vi "BRig_RT__Case_Exp__State_initTrial__LC_Cue__v10.vi"(6 "input_arrTrig":bool[](array[boolean]), 8 "input_dataTrial":u16[][](array[numeric]), 9 "input_dataExp":u16[](array[numeric]), 10 "input_dataLC":u16[](array[numeric]), 11 "input_dataCurrent":u16[](array[numeric])) -> (0 "output_dataTrial":u16[][](array[numeric]), 3 "output_dataCurrent":u16[](array[numeric]), 4 "output_arrTrig":bool[](array[boolean]))   [LabVIEW 2014]
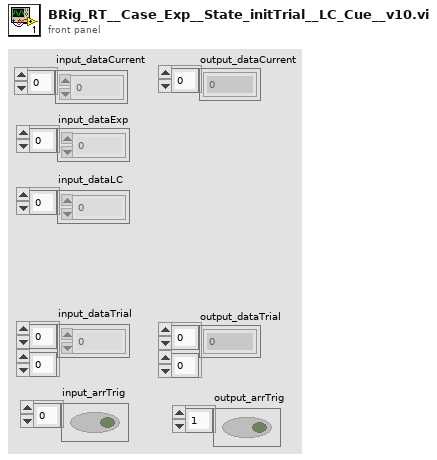
[diagram p1: front panel]
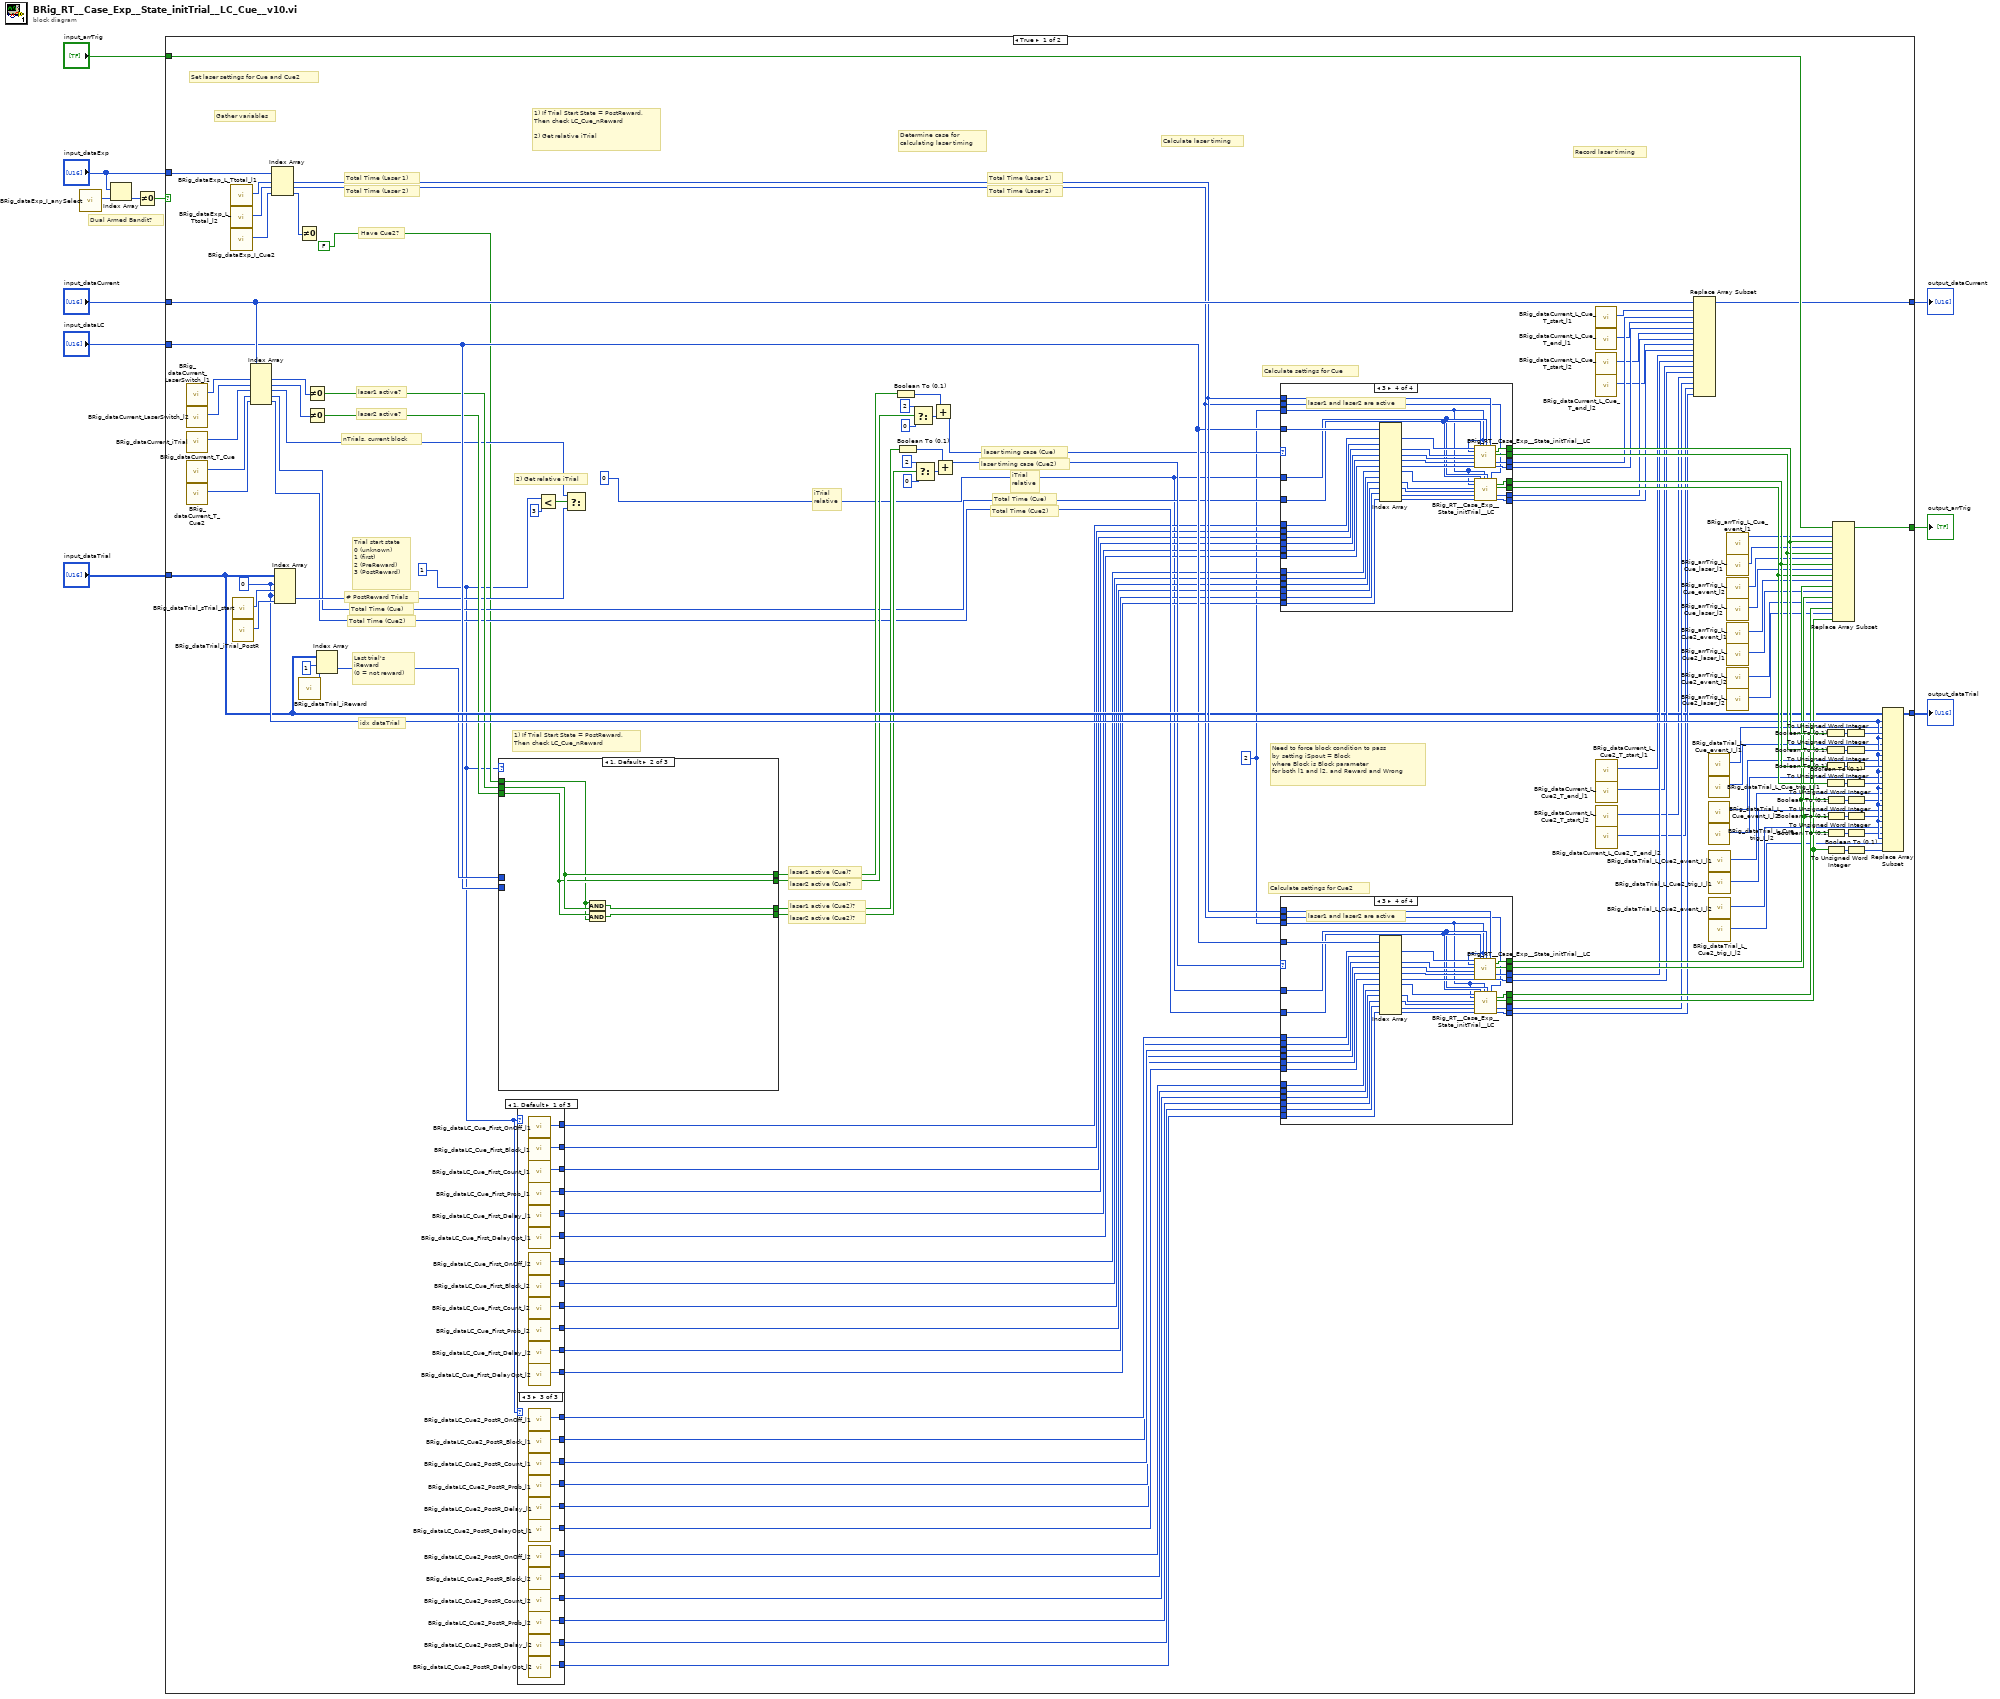
[diagram p0: block diagram]
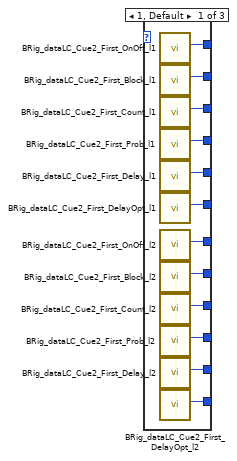
[diagram p2: hidden frame]
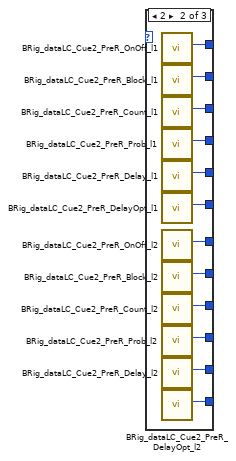
[diagram p3: hidden frame]
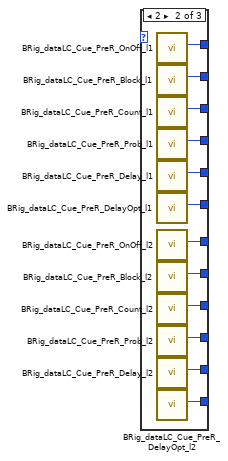
[diagram p4: hidden frame]
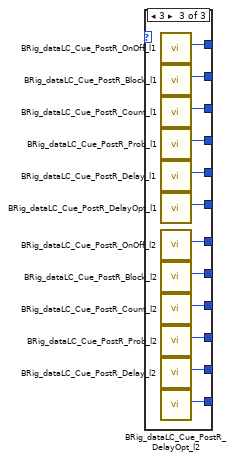
[diagram p5: hidden frame]
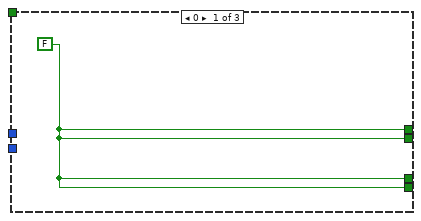
[diagram p6: hidden frame]
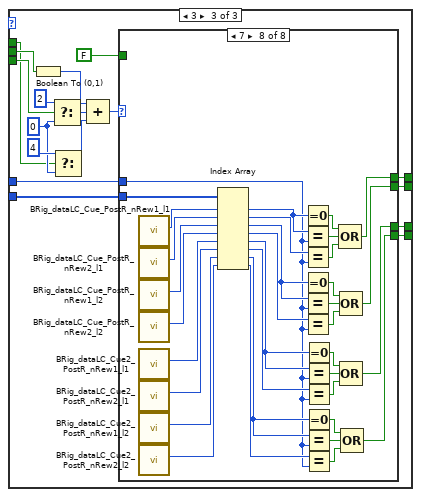
[diagram p7: hidden frame]
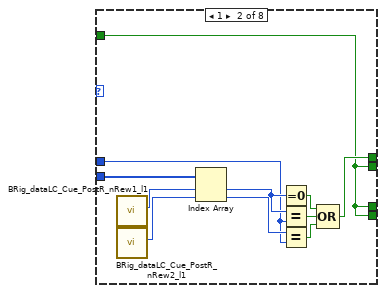
[diagram p9: hidden frame]
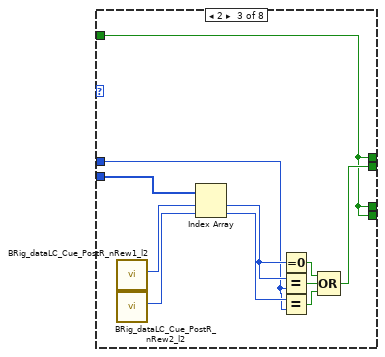
[diagram p10: hidden frame]
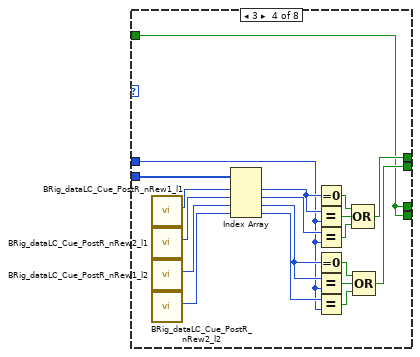
[diagram p11: hidden frame]
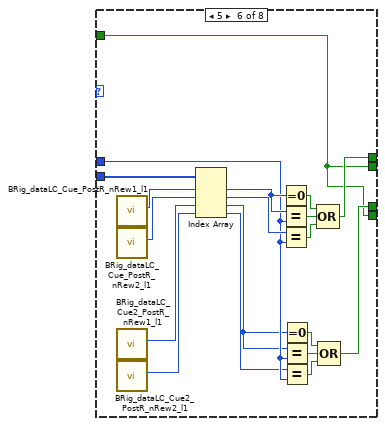
[diagram p13: hidden frame]
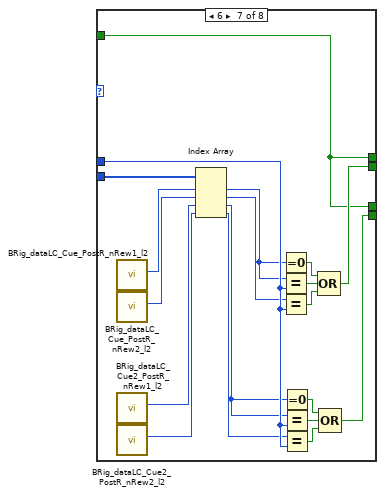
[diagram p14: hidden frame]
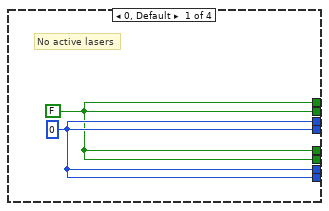
[diagram p15: hidden frame]
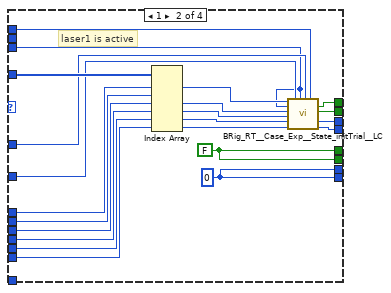
[diagram p16: hidden frame]
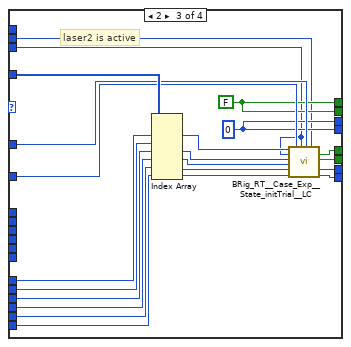
[diagram p17: hidden frame]
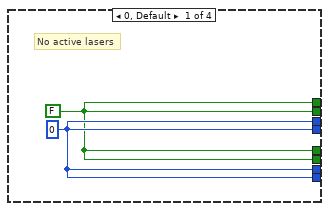
[diagram p18: hidden frame]
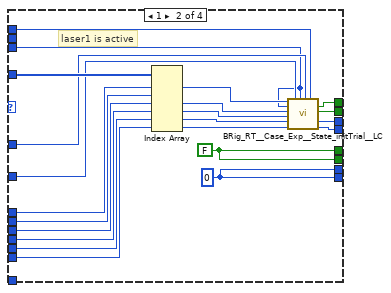
[diagram p19: hidden frame]
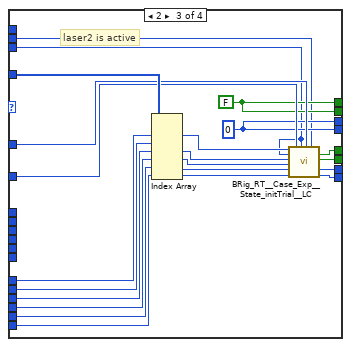
[diagram p20: hidden frame]
diagram:
  # "Dual Armed Bandit?"
  n1 = call "BRig_dataExp_I_anySelect.vi"() -> ("output_I_anySelect"=w4:i32)  [unwired: 11 in]
  n2 = Index Array(array="input_dataExp", index=w4) -> (element=w3:u16)
  n3 = Not Equal To 0?(x=w3) -> (x != 0?=w1:bool)
  n4 = case shown="True" w1 {
    tunnel: "input_arrTrig" -> [w135 w642]
    tunnel: [w134 w641] -> w10
    tunnel: [w121 w628] -> w9
    tunnel: "input_dataCurrent" -> [w120 w627]
    tunnel: [w119 w626] -> w7
    tunnel: "input_dataExp" -> [w112 w619]
    tunnel: "input_dataTrial" -> [w86 w592]
    tunnel: "input_dataLC" -> [w84 w590]
    frame True {
      w12 = u16 2 ("input_sState_start")
      w13 = u16 1
      w14 = u16 0
      w105 = 0
      # "Need to force block condition to pass\nby setting iSpout = Block\nwhere Block is Block parameter\nfor both l1 and l2, and Reward and Wrong"
      # "Record laser timing"
      # "Calculate laser timing"
      # "Total Time (Cue2)"
      # "Total Time (Cue)"
      # "iTrial\nrelative"
      # "Total Time (Laser 2)"
      # "Total Time (Laser 1)"
      # "laser timing case (Cue2)"
      # "Determine case for\ncalculating laser timing"
      # "2) Get relative iTrial"
      # "1) If Trial Start State = PostReward,\nThen check LC_Cue_nReward"
      # "laser2 active (Cue2)?"
      # "laser1 active (Cue2)?"
      # "laser2 active (Cue)?"
      # "laser1 active (Cue)?"
      # "1) If Trial Start State = PostReward,\nThen check LC_Cue_nReward\n\n2) Get relative iTrial"
      # "Gather variables"
      # "Last trial's\niReward\n(0 = not reward)"
      # "nTrials, current block"
      # "idx dataTrial"
      # "Total Time (Cue2)"
      # "Total Time (Cue)"
      # "# PostReward Trials"
      # "Have Cue2?"
      # "Total Time (Laser 2)"
      # "Total Time (Laser 1)"
      # "Calculate settings for Cue2"
      # "Calculate settings for Cue"
      # "Set laser settings for Cue and Cue2"
      # "iTrial\nrelative"
      # "laser timing case (Cue)"
      # "Trial start state\n0 (unknown)\n1 (first)\n2 (PreReward)\n3 (PostReward)"
      # "laser2 active?"
      # "laser1 active?"
      n5 = call "BRig_dataCurrent_LaserSwitch_l1.vi"() -> ("output_LaserSwitch_l1"=w144:i32)  [unwired: 11 in]
      n6 = call "BRig_dataCurrent_LaserSwitch_l2.vi"() -> ("output_LaserSwitch_l2"=w143:i32)  [unwired: 11 in]
      n7 = call "BRig_dataCurrent_iTrial.vi"() -> ("output_iTrial"=w110:i32)  [unwired: 11 in]
      n8 = call "BRig_dataCurrent_T_Cue.vi"() -> ("output_T_Cue"=w67:i32)  [unwired: 11 in]
      n9 = call "BRig_dataCurrent_T_Cue2.vi"() -> ("output_T_Cue2"=w66:i32)  [unwired: 11 in]
      n10 = call "BRig_dataExp_L_Ttotal_l1.vi"() -> ("output_L_Ttotal_l1"=w113:i32)  [unwired: 11 in]
      n11 = call "BRig_dataExp_L_Ttotal_l2.vi"() -> ("output_L_Ttotal_l2"=w114:i32)  [unwired: 11 in]
      n12 = call "BRig_dataExp_I_Cue2.vi"() -> ("output_I_Cue2"=w90:i32)  [unwired: 11 in]
      n13 = call "BRig_dataTrial_sTrial_start.vi"() -> ("output_sTrial_start"=w140:i32)  [unwired: 11 in]
      n14 = call "BRig_dataTrial_iTrial_PostR.vi"() -> ("output_iTrial_PostR"=w111:i32)  [unwired: 11 in]
      n15 = Index Array(array=w120, index #1=w144, index #2=w143, index #3=w110, index #4=w67, index #5=w66) -> (element #1=w142:u16, element #2=w141:u16, element #3=w79:u16, element #4=w65:u16, element #5=w64:u16)
      n16 = Index Array(array=w112, index #1=w113, index #2=w114, index #3=w90) -> (element #1=w100:u16, element #2=w99:u16, element #3=w89:u16)
      n17 = Index Array(array=w86, index (row) #1=w105, index (col) #1=w140, index (row) #2=w105, index (col) #2=w111) -> (element #2=w78:u16)  [unwired: 1 out]
      n18 = Not Equal To 0?(x=w89) -> ()  [unwired: 1 out]
      n19 = call "BRig_dataTrial_iReward.vi"() -> ("output_iReward"=w87:i32)  [unwired: 11 in]
      n20 = Not Equal To 0?(x=w142) -> (x != 0?=w82:bool)
      n21 = Not Equal To 0?(x=w141) -> (x != 0?=w83:bool)
      n22 = Index Array(array=w86, index (row)=1 ("disabled index (row)"), index (col)=w87) -> (element=w85:u16)
      n23 = case shown="1, Default" w13 {
        tunnel: w85 -> [_ _ w231]
        tunnel: w84 -> [_ _ w232]
        tunnel: w83 -> [_ w221 w224]
        tunnel: w82 -> [_ w222 w225]
        tunnel: FALSE -> [_ w220 w223]
        tunnel: [w217 w222 w230] -> w77
        tunnel: [w217 w221 w229] -> w76
        tunnel: [w217 w219 w228] -> w71
        tunnel: [w217 w218 w227] -> w70
        frame 0 {
          w217 = FALSE
        }
        frame 1, Default {
          n24 = And(x=w220, y=w222) -> (x .and. y?=w219:bool)
          n25 = And(x=w221, y=w220) -> (x .and. y?=w218:bool)
        }
        frame 3 {
          w237 = i16 0 ("f")
          n26 = Boolean To (0,1)(Boolean=w225) -> (0, 1=w235:i16)
          n27 = Select(t=i16 2, s=w224, f=w237) -> (s? t:f=w236:i16)
          n28 = Select(t=i16 4, s=w223, f=w237) -> (s? t:f=w234:i16)
          n29 = Compound Arithmetic op=ADD(w235, w236, w234) -> (w233:i16)
          n30 = case shown="7" w233 {
            tunnel: w232 -> [_ w246 w257 w271 _ w296 w317 w344]
            tunnel: w231 -> [_ w245 w256 w270 _ w292 w313 w333]
            tunnel: [w240 w244 w254 w269 w282 w291 w310 w332] -> w230
            tunnel: [w240 w243 w255 w268 w282 w289 w312 w331] -> w229
            tunnel: [w240 w243 w254 w267 w282 w290 w310 w330] -> w228
            tunnel: [w240 w243 w254 w267 w282 w289 w311 w329] -> w227
            tunnel: FALSE -> [w240 w243 w254 w267 w282 w289 w310 _]
            frame 0, Default {
            }
            frame 1 {
              n31 = call "BRig_dataLC_Cue_PostR_nRew1_l1.vi"() -> ("output_Cue_PostR_nRew1_l1"=w241:i32)  [unwired: 11 in]
              n32 = call "BRig_dataLC_Cue_PostR_nRew2_l1.vi"() -> ("output_Cue_PostR_nRew2_l1"=w242:i32)  [unwired: 11 in]
              n33 = Index Array(array=w246, index #1=w241, index #2=w242) -> (element #1=w248:u16, element #2=w247:u16)
              n34 = Equal To 0?(x=w248) -> (x = 0?=w249:bool)
              n35 = Equal?(x=w248, y=w245) -> (x = y?=w250:bool)
              n36 = Equal?(x=w247, y=w245) -> (x = y?=w251:bool)
              n37 = Compound Arithmetic op=OR(w249, w250, w251) -> (w244:bool)
            }
            frame 2 {
              n38 = call "BRig_dataLC_Cue_PostR_nRew1_l2.vi"() -> ("output_Cue_PostR_nRew1_l2"=w252:i32)  [unwired: 11 in]
              n39 = call "BRig_dataLC_Cue_PostR_nRew2_l2.vi"() -> ("output_Cue_PostR_nRew2_l2"=w253:i32)  [unwired: 11 in]
              n40 = Index Array(array=w257, index #1=w252, index #2=w253) -> (element #1=w258:u16, element #2=w259:u16)
              n41 = Equal To 0?(x=w258) -> (x = 0?=w261:bool)
              n42 = Equal?(x=w258, y=w256) -> (x = y?=w260:bool)
              n43 = Equal?(x=w259, y=w256) -> (x = y?=w262:bool)
              n44 = Compound Arithmetic op=OR(w261, w260, w262) -> (w255:bool)
            }
            frame 3 {
              n45 = call "BRig_dataLC_Cue_PostR_nRew1_l1.vi"() -> ("output_Cue_PostR_nRew1_l1"=w263:i32)  [unwired: 11 in]
              n46 = call "BRig_dataLC_Cue_PostR_nRew2_l1.vi"() -> ("output_Cue_PostR_nRew2_l1"=w264:i32)  [unwired: 11 in]
              n47 = call "BRig_dataLC_Cue_PostR_nRew1_l2.vi"() -> ("output_Cue_PostR_nRew1_l2"=w265:i32)  [unwired: 11 in]
              n48 = call "BRig_dataLC_Cue_PostR_nRew2_l2.vi"() -> ("output_Cue_PostR_nRew2_l2"=w266:i32)  [unwired: 11 in]
              n49 = Index Array(array=w271, index #1=w263, index #2=w264, index #3=w265, index #4=w266) -> (element #1=w275:u16, element #2=w274:u16, element #3=w272:u16, element #4=w273:u16)
              n50 = Equal To 0?(x=w275) -> (x = 0?=w276:bool)
              n51 = Equal?(x=w275, y=w270) -> (x = y?=w277:bool)
              n52 = Equal?(x=w274, y=w270) -> (x = y?=w278:bool)
              n53 = Equal To 0?(x=w272) -> (x = 0?=w280:bool)
              n54 = Equal?(x=w272, y=w270) -> (x = y?=w279:bool)
              n55 = Equal?(x=w273, y=w270) -> (x = y?=w281:bool)
              n56 = Compound Arithmetic op=OR(w276, w277, w278) -> (w269:bool)
              n57 = Compound Arithmetic op=OR(w280, w279, w281) -> (w268:bool)
            }
            frame 4 {
            }
            frame 5 {
              n58 = call "BRig_dataLC_Cue_PostR_nRew1_l1.vi"() -> ("output_Cue_PostR_nRew1_l1"=w285:i32)  [unwired: 11 in]
              n59 = call "BRig_dataLC_Cue_PostR_nRew2_l1.vi"() -> ("output_Cue_PostR_nRew2_l1"=w286:i32)  [unwired: 11 in]
              n60 = call "BRig_dataLC_Cue2_PostR_nRew1_l1.vi"() -> ("output_Cue2_PostR_nRew1_l1"=w283:i32)  [unwired: 11 in]
              n61 = call "BRig_dataLC_Cue2_PostR_nRew2_l1.vi"() -> ("output_Cue2_PostR_nRew2_l1"=w284:i32)  [unwired: 11 in]
              n62 = Index Array(array=w296, index #1=w285, index #2=w286, index #3=w283, index #4=w284) -> (element #1=w298:u16, element #2=w297:u16, element #3=w288:u16, element #4=w287:u16)
              n63 = Equal To 0?(x=w298) -> (x = 0?=w299:bool)
              n64 = Equal?(x=w298, y=w292) -> (x = y?=w300:bool)
              n65 = Equal?(x=w297, y=w292) -> (x = y?=w301:bool)
              n66 = Equal To 0?(x=w288) -> (x = 0?=w295:bool)
              n67 = Equal?(x=w288, y=w292) -> (x = y?=w294:bool)
              n68 = Equal?(x=w287, y=w292) -> (x = y?=w293:bool)
              n69 = Compound Arithmetic op=OR(w299, w300, w301) -> (w291:bool)
              n70 = Compound Arithmetic op=OR(w295, w294, w293) -> (w290:bool)
            }
            frame 6 {
              n71 = call "BRig_dataLC_Cue_PostR_nRew1_l2.vi"() -> ("output_Cue_PostR_nRew1_l2"=w305:i32)  [unwired: 11 in]
              n72 = call "BRig_dataLC_Cue_PostR_nRew2_l2.vi"() -> ("output_Cue_PostR_nRew2_l2"=w304:i32)  [unwired: 11 in]
              n73 = call "BRig_dataLC_Cue2_PostR_nRew1_l2.vi"() -> ("output_Cue2_PostR_nRew1_l2"=w303:i32)  [unwired: 11 in]
              n74 = call "BRig_dataLC_Cue2_PostR_nRew2_l2.vi"() -> ("output_Cue2_PostR_nRew2_l2"=w302:i32)  [unwired: 11 in]
              n75 = Index Array(array=w317, index #1=w305, index #2=w304, index #3=w303, index #4=w302) -> (element #1=w309:u16, element #2=w308:u16, element #3=w307:u16, element #4=w306:u16)
              n76 = Equal To 0?(x=w309) -> (x = 0?=w319:bool)
              n77 = Equal?(x=w309, y=w313) -> (x = y?=w318:bool)
              n78 = Equal?(x=w308, y=w313) -> (x = y?=w320:bool)
              n79 = Equal To 0?(x=w307) -> (x = 0?=w315:bool)
              n80 = Equal?(x=w307, y=w313) -> (x = y?=w316:bool)
              n81 = Equal?(x=w306, y=w313) -> (x = y?=w314:bool)
              n82 = Compound Arithmetic op=OR(w319, w318, w320) -> (w312:bool)
              n83 = Compound Arithmetic op=OR(w315, w316, w314) -> (w311:bool)
            }
            frame 7 {
              n84 = call "BRig_dataLC_Cue_PostR_nRew1_l1.vi"() -> ("output_Cue_PostR_nRew1_l1"=w325:i32)  [unwired: 11 in]
              n85 = call "BRig_dataLC_Cue_PostR_nRew2_l1.vi"() -> ("output_Cue_PostR_nRew2_l1"=w326:i32)  [unwired: 11 in]
              n86 = call "BRig_dataLC_Cue_PostR_nRew1_l2.vi"() -> ("output_Cue_PostR_nRew1_l2"=w327:i32)  [unwired: 11 in]
              n87 = call "BRig_dataLC_Cue_PostR_nRew2_l2.vi"() -> ("output_Cue_PostR_nRew2_l2"=w328:i32)  [unwired: 11 in]
              n88 = call "BRig_dataLC_Cue2_PostR_nRew1_l1.vi"() -> ("output_Cue2_PostR_nRew1_l1"=w324:i32)  [unwired: 11 in]
              n89 = call "BRig_dataLC_Cue2_PostR_nRew2_l1.vi"() -> ("output_Cue2_PostR_nRew2_l1"=w323:i32)  [unwired: 11 in]
              n90 = call "BRig_dataLC_Cue2_PostR_nRew1_l2.vi"() -> ("output_Cue2_PostR_nRew1_l2"=w322:i32)  [unwired: 11 in]
              n91 = call "BRig_dataLC_Cue2_PostR_nRew2_l2.vi"() -> ("output_Cue2_PostR_nRew2_l2"=w321:i32)  [unwired: 11 in]
              n92 = Index Array(array=w344, index #1=w325, index #2=w326, index #3=w327, index #4=w328, index #5=w324, index #6=w323, index #7=w322, index #8=w321) -> (element #1=w348:u16, element #2=w347:u16, element #3=w345:u16, element #4=w346:u16, element #5=w337:u16, element #6=w336:u16, element #7=w334:u16, element #8=w335:u16)
              n93 = Equal To 0?(x=w348) -> (x = 0?=w349:bool)
              n94 = Equal?(x=w348, y=w333) -> (x = y?=w350:bool)
              n95 = Equal?(x=w347, y=w333) -> (x = y?=w351:bool)
              n96 = Equal To 0?(x=w345) -> (x = 0?=w353:bool)
              n97 = Equal?(x=w345, y=w333) -> (x = y?=w352:bool)
              n98 = Equal?(x=w346, y=w333) -> (x = y?=w354:bool)
              n99 = Equal To 0?(x=w337) -> (x = 0?=w343:bool)
              n100 = Equal?(x=w337, y=w333) -> (x = y?=w342:bool)
              n101 = Equal?(x=w336, y=w333) -> (x = y?=w341:bool)
              n102 = Equal To 0?(x=w334) -> (x = 0?=w339:bool)
              n103 = Equal?(x=w334, y=w333) -> (x = y?=w340:bool)
              n104 = Equal?(x=w335, y=w333) -> (x = y?=w338:bool)
              n105 = Compound Arithmetic op=OR(w349, w350, w351) -> (w332:bool)
              n106 = Compound Arithmetic op=OR(w353, w352, w354) -> (w331:bool)
              n107 = Compound Arithmetic op=OR(w343, w342, w341) -> (w330:bool)
              n108 = Compound Arithmetic op=OR(w339, w340, w338) -> (w329:bool)
            }
          }
        }
      }
      n109 = case shown="1, Default" w13 {
        tunnel: [w181 w204 w215] -> w52
        tunnel: [w182 w193 w214] -> w53
        tunnel: [w183 w194 w213] -> w54
        tunnel: [w184 w195 w212] -> w55
        tunnel: [w185 w196 w211] -> w56
        tunnel: [w186 w197 w210] -> w57
        tunnel: [w187 w203 w209] -> w58
        tunnel: [w188 w198 w208] -> w59
        tunnel: [w189 w199 w207] -> w60
        tunnel: [w190 w200 w206] -> w61
        tunnel: [w191 w201 w205] -> w62
        tunnel: [w192 w202 w216] -> w63
        frame 1, Default {
          n110 = call "BRig_dataLC_Cue_First_OnOff_l1.vi"() -> ("output_Cue_First_OnOff"=w181:i32)  [unwired: 11 in]
          n111 = call "BRig_dataLC_Cue_First_Block_l1.vi"() -> ("output_Cue_First_Block"=w182:i32)  [unwired: 11 in]
          n112 = call "BRig_dataLC_Cue_First_Count_l1.vi"() -> ("output_Cue_First_Count"=w183:i32)  [unwired: 11 in]
          n113 = call "BRig_dataLC_Cue_First_Prob_l1.vi"() -> ("output_Cue_First_Prob"=w184:i32)  [unwired: 11 in]
          n114 = call "BRig_dataLC_Cue_First_Delay_l1.vi"() -> ("output_Cue_First_Delay"=w185:i32)  [unwired: 11 in]
          n115 = call "BRig_dataLC_Cue_First_DelayOpt_l1.vi"() -> ("output_Cue_First_DelayOpt"=w186:i32)  [unwired: 11 in]
          n116 = call "BRig_dataLC_Cue_First_OnOff_l2.vi"() -> ("output_Cue_First_OnOff_l2"=w187:i32)  [unwired: 11 in]
          n117 = call "BRig_dataLC_Cue_First_Block_l2.vi"() -> ("output_Cue_First_Block_l2"=w188:i32)  [unwired: 11 in]
          n118 = call "BRig_dataLC_Cue_First_Count_l2.vi"() -> ("output_Cue_First_Count_l2"=w189:i32)  [unwired: 11 in]
          n119 = call "BRig_dataLC_Cue_First_Prob_l2.vi"() -> ("output_Cue_First_Prob_l2"=w190:i32)  [unwired: 11 in]
          n120 = call "BRig_dataLC_Cue_First_Delay_l2.vi"() -> ("output_Cue_First_Delay_l2"=w191:i32)  [unwired: 11 in]
          n121 = call "BRig_dataLC_Cue_First_DelayOpt_l2.vi"() -> ("output_Cue_First_DelayOpt_l2"=w192:i32)  [unwired: 11 in]
        }
        frame 2 {
          n122 = call "BRig_dataLC_Cue_PreR_OnOff_l1.vi"() -> ("output_Cue_PreR_OnOff"=w204:i32)  [unwired: 11 in]
          n123 = call "BRig_dataLC_Cue_PreR_Block_l1.vi"() -> ("output_Cue_PreR_Block"=w193:i32)  [unwired: 11 in]
          n124 = call "BRig_dataLC_Cue_PreR_Count_l1.vi"() -> ("output_Cue_PreR_Count"=w194:i32)  [unwired: 11 in]
          n125 = call "BRig_dataLC_Cue_PreR_Prob_l1.vi"() -> ("output_Cue_PreR_Prob"=w195:i32)  [unwired: 11 in]
          n126 = call "BRig_dataLC_Cue_PreR_Delay_l1.vi"() -> ("output_Cue_PreR_Delay"=w196:i32)  [unwired: 11 in]
          n127 = call "BRig_dataLC_Cue_PreR_DelayOpt_l1.vi"() -> ("output_Cue_PreR_DelayOpt"=w197:i32)  [unwired: 11 in]
          n128 = call "BRig_dataLC_Cue_PreR_OnOff_l2.vi"() -> ("output_Cue_PreR_OnOff_l2"=w203:i32)  [unwired: 11 in]
          n129 = call "BRig_dataLC_Cue_PreR_Block_l2.vi"() -> ("output_Cue_PreR_Block_l2"=w198:i32)  [unwired: 11 in]
          n130 = call "BRig_dataLC_Cue_PreR_Count_l2.vi"() -> ("output_Cue_PreR_Count_l2"=w199:i32)  [unwired: 11 in]
          n131 = call "BRig_dataLC_Cue_PreR_Prob_l2.vi"() -> ("output_Cue_PreR_Prob_l2"=w200:i32)  [unwired: 11 in]
          n132 = call "BRig_dataLC_Cue_PreR_Delay_l2.vi"() -> ("output_Cue_PreR_Delay_l2"=w201:i32)  [unwired: 11 in]
          n133 = call "BRig_dataLC_Cue_PreR_DelayOpt_l2.vi"() -> ("output_Cue_PreR_DelayOpt_l2"=w202:i32)  [unwired: 11 in]
        }
        frame 3 {
          n134 = call "BRig_dataLC_Cue_PostR_OnOff_l1.vi"() -> ("output_Cue_PostR_OnOff"=w215:i32)  [unwired: 11 in]
          n135 = call "BRig_dataLC_Cue_PostR_Block_l1.vi"() -> ("output_Cue_PostR_Block"=w214:i32)  [unwired: 11 in]
          n136 = call "BRig_dataLC_Cue_PostR_Count_l1.vi"() -> ("output_Cue_PostR_Count"=w213:i32)  [unwired: 11 in]
          n137 = call "BRig_dataLC_Cue_PostR_Prob_l1.vi"() -> ("output_Cue_PostR_Prob"=w212:i32)  [unwired: 11 in]
          n138 = call "BRig_dataLC_Cue_PostR_Delay_l1.vi"() -> ("output_Cue_PostR_Delay"=w211:i32)  [unwired: 11 in]
          n139 = call "BRig_dataLC_Cue_PostR_DelayOpt_l1.vi"() -> ("output_Cue_PostR_DelayOpt"=w210:i32)  [unwired: 11 in]
          n140 = call "BRig_dataLC_Cue_PostR_OnOff_l2.vi"() -> ("output_Cue_PostR_OnOff_l2"=w209:i32)  [unwired: 11 in]
          n141 = call "BRig_dataLC_Cue_PostR_Block_l2.vi"() -> ("output_Cue_PostR_Block_l2"=w208:i32)  [unwired: 11 in]
          n142 = call "BRig_dataLC_Cue_PostR_Count_l2.vi"() -> ("output_Cue_PostR_Count_l2"=w207:i32)  [unwired: 11 in]
          n143 = call "BRig_dataLC_Cue_PostR_Prob_l2.vi"() -> ("output_Cue_PostR_Prob_l2"=w206:i32)  [unwired: 11 in]
          n144 = call "BRig_dataLC_Cue_PostR_Delay_l2.vi"() -> ("output_Cue_PostR_Delay_l2"=w205:i32)  [unwired: 11 in]
          n145 = call "BRig_dataLC_Cue_PostR_DelayOpt_l2.vi"() -> ("output_Cue_PostR_DelayOpt_l2"=w216:i32)  [unwired: 11 in]
        }
      }
      n146 = case shown="3" w13 {
        tunnel: [w156 w168 w180] -> w51
        tunnel: [w155 w167 w179] -> w50
        tunnel: [w154 w166 w178] -> w49
        tunnel: [w153 w165 w177] -> w48
        tunnel: [w152 w164 w176] -> w47
        tunnel: [w151 w163 w175] -> w46
        tunnel: [w150 w162 w174] -> w45
        tunnel: [w149 w161 w173] -> w44
        tunnel: [w148 w160 w172] -> w43
        tunnel: [w147 w159 w171] -> w42
        tunnel: [w146 w158 w170] -> w41
        tunnel: [w145 w157 w169] -> w40
        frame 1, Default {
          n147 = call "BRig_dataLC_Cue2_First_OnOff_l1.vi"() -> ("output_Cue2_First_OnOff"=w156:i32)  [unwired: 11 in]
          n148 = call "BRig_dataLC_Cue2_First_Block_l1.vi"() -> ("output_Cue2_First_Block"=w155:i32)  [unwired: 11 in]
          n149 = call "BRig_dataLC_Cue2_First_Count_l1.vi"() -> ("output_Cue2_First_Count"=w154:i32)  [unwired: 11 in]
          n150 = call "BRig_dataLC_Cue2_First_Prob_l1.vi"() -> ("output_Cue2_First_Prob"=w153:i32)  [unwired: 11 in]
          n151 = call "BRig_dataLC_Cue2_First_Delay_l1.vi"() -> ("output_Cue2_First_Delay"=w152:i32)  [unwired: 11 in]
          n152 = call "BRig_dataLC_Cue2_First_DelayOpt_l1.vi"() -> ("output_Cue2_First_DelayOpt"=w151:i32)  [unwired: 11 in]
          n153 = call "BRig_dataLC_Cue2_First_OnOff_l2.vi"() -> ("output_Cue2_First_OnOff_l2"=w150:i32)  [unwired: 11 in]
          n154 = call "BRig_dataLC_Cue2_First_Block_l2.vi"() -> ("output_Cue2_First_Block_l2"=w149:i32)  [unwired: 11 in]
          n155 = call "BRig_dataLC_Cue2_First_Count_l2.vi"() -> ("output_Cue2_First_Count_l2"=w148:i32)  [unwired: 11 in]
          n156 = call "BRig_dataLC_Cue2_First_Prob_l2.vi"() -> ("output_Cue2_First_Prob_l2"=w147:i32)  [unwired: 11 in]
          n157 = call "BRig_dataLC_Cue2_First_Delay_l2.vi"() -> ("output_Cue2_First_Delay_l2"=w146:i32)  [unwired: 11 in]
          n158 = call "BRig_dataLC_Cue2_First_DelayOpt_l2.vi"() -> ("output_Cue2_First_DelayOpt_l2"=w145:i32)  [unwired: 11 in]
        }
        frame 2 {
          n159 = call "BRig_dataLC_Cue2_PreR_OnOff_l1.vi"() -> ("output_Cue2_PreR_OnOff"=w168:i32)  [unwired: 11 in]
          n160 = call "BRig_dataLC_Cue2_PreR_Block_l1.vi"() -> ("output_Cue2_PreR_Block"=w167:i32)  [unwired: 11 in]
          n161 = call "BRig_dataLC_Cue2_PreR_Count_l1.vi"() -> ("output_Cue2_PreR_Count"=w166:i32)  [unwired: 11 in]
          n162 = call "BRig_dataLC_Cue2_PreR_Prob_l1.vi"() -> ("output_Cue2_PreR_Prob"=w165:i32)  [unwired: 11 in]
          n163 = call "BRig_dataLC_Cue2_PreR_Delay_l1.vi"() -> ("output_Cue2_PreR_Delay"=w164:i32)  [unwired: 11 in]
          n164 = call "BRig_dataLC_Cue2_PreR_DelayOpt_l1.vi"() -> ("output_Cue2_PreR_DelayOpt"=w163:i32)  [unwired: 11 in]
          n165 = call "BRig_dataLC_Cue2_PreR_OnOff_l2.vi"() -> ("output_Cue2_PreR_OnOff_l2"=w162:i32)  [unwired: 11 in]
          n166 = call "BRig_dataLC_Cue2_PreR_Block_l2.vi"() -> ("output_Cue2_PreR_Block_l2"=w161:i32)  [unwired: 11 in]
          n167 = call "BRig_dataLC_Cue2_PreR_Count_l2.vi"() -> ("output_Cue2_PreR_Count_l2"=w160:i32)  [unwired: 11 in]
          n168 = call "BRig_dataLC_Cue2_PreR_Prob_l2.vi"() -> ("output_Cue2_PreR_Prob_l2"=w159:i32)  [unwired: 11 in]
          n169 = call "BRig_dataLC_Cue2_PreR_Delay_l2.vi"() -> ("output_Cue2_PreR_Delay_l2"=w158:i32)  [unwired: 11 in]
          n170 = call "BRig_dataLC_Cue2_PreR_DelayOpt_l2.vi"() -> ("output_Cue2_PreR_DelayOpt_l2"=w157:i32)  [unwired: 11 in]
        }
        frame 3 {
          n171 = call "BRig_dataLC_Cue2_PostR_OnOff_l1.vi"() -> ("output_Cue2_PostR_OnOff"=w180:i32)  [unwired: 11 in]
          n172 = call "BRig_dataLC_Cue2_PostR_Block_l1.vi"() -> ("output_Cue2_PostR_Block"=w179:i32)  [unwired: 11 in]
          n173 = call "BRig_dataLC_Cue2_PostR_Count_l1.vi"() -> ("output_Cue2_PostR_Count"=w178:i32)  [unwired: 11 in]
          n174 = call "BRig_dataLC_Cue2_PostR_Prob_l1.vi"() -> ("output_Cue2_PostR_Prob"=w177:i32)  [unwired: 11 in]
          n175 = call "BRig_dataLC_Cue2_PostR_Delay_l1.vi"() -> ("output_Cue2_PostR_Delay"=w176:i32)  [unwired: 11 in]
          n176 = call "BRig_dataLC_Cue2_PostR_DelayOpt_l1.vi"() -> ("output_Cue2_PostR_DelayOpt"=w175:i32)  [unwired: 11 in]
          n177 = call "BRig_dataLC_Cue2_PostR_OnOff_l2.vi"() -> ("output_Cue2_PostR_OnOff_l2"=w174:i32)  [unwired: 11 in]
          n178 = call "BRig_dataLC_Cue2_PostR_Block_l2.vi"() -> ("output_Cue2_PostR_Block_l2"=w173:i32)  [unwired: 11 in]
          n179 = call "BRig_dataLC_Cue2_PostR_Count_l2.vi"() -> ("output_Cue2_PostR_Count_l2"=w172:i32)  [unwired: 11 in]
          n180 = call "BRig_dataLC_Cue2_PostR_Prob_l2.vi"() -> ("output_Cue2_PostR_Prob_l2"=w171:i32)  [unwired: 11 in]
          n181 = call "BRig_dataLC_Cue2_PostR_Delay_l2.vi"() -> ("output_Cue2_PostR_Delay_l2"=w170:i32)  [unwired: 11 in]
          n182 = call "BRig_dataLC_Cue2_PostR_DelayOpt_l2.vi"() -> ("output_Cue2_PostR_DelayOpt_l2"=w169:i32)  [unwired: 11 in]
        }
      }
      n183 = Less?(x=w13, y=u16 3) -> (x < y?=w80:bool)
      n184 = Select(t=w79, s=w80, f=w78) -> ()  [unwired: 1 out]
      n185 = Boolean To (0,1)(Boolean=w77) -> (0, 1=w137:i16)
      n186 = Boolean To (0,1)(Boolean=w71) -> (0, 1=w74:i16)
      n187 = Select(t=i16 2, s=w76, f=i16 0) -> (s? t:f=w138:i16)
      n188 = Select(t=i16 2, s=w70, f=i16 0) -> (s? t:f=w73:i16)
      n189 = Add(x=w137, y=w138) -> (x+y=w69:i16)
      n190 = Add(x=w74, y=w73) -> (x+y=w68:i16)
      n191 = case shown="3" w69 {
        tunnel: w84 -> [_ w460 w482 w518]
        tunnel: w12 -> [_ w439 w461 w483]
        tunnel: w65 -> [_ w454 w476 w507]
        tunnel: w14 -> [_ w453 w475 w506]
        tunnel: [w437 w452 w464 w505] -> w129
        tunnel: [w437 w451 w464 w504] -> w126
        tunnel: [w438 w450 w463 w503] -> w118
        tunnel: [w438 w449 w463 w502] -> w117
        tunnel: [w437 w442 w474 w501] -> w122
        tunnel: [w438 w441 w473 w500] -> w116
        tunnel: [w437 w442 w472 w499] -> w124
        tunnel: [w438 w441 w471 w498] -> w115
        tunnel: w52 -> [_ w448 _ w497]
        tunnel: w53 -> [_ w447 _ w496]
        tunnel: w54 -> [_ w446 _ w495]
        tunnel: w55 -> [_ w445 _ w494]
        tunnel: w56 -> [_ w444 _ w493]
        tunnel: w57 -> [_ w443 _ w492]
        tunnel: w58 -> [_ _ w470 w491]
        tunnel: w59 -> [_ _ w469 w490]
        tunnel: w60 -> [_ _ w468 w489]
        tunnel: w61 -> [_ _ w467 w488]
        tunnel: w62 -> [_ _ w466 w487]
        tunnel: w63 -> [_ _ w465 w486]
        tunnel: w100 -> [_ w440 _ w485]
        tunnel: w99 -> [_ _ w462 w484]
        frame 0, Default {
          w438 = u16 0
          w437 = FALSE
          # "No active lasers"
        }
        frame 1 {
          w441 = u16 0
          w442 = FALSE
          # "laser1 is active"
          n192 = Index Array(array=w460, index #1=w448, index #2=w447, index #3=w446, index #4=w445, index #5=w444, index #6=w443) -> (element #1=w459:u16, element #3=w458:u16, element #4=w457:u16, element #5=w456:u16, element #6=w455:u16)  [unwired: 1 out]
          n193 = call "BRig_RT__Case_Exp__State_initTrial__LC.vi"("input_L_OnOff"=w459, "input_L_Block"=w439, "input_L_Count"=w458, "input_L_Prob"=w457, "input_L_Tdelay"=w456, "input_L_delayOpt"=w455, "input_T_state"=w454, "input_iSpout"=w439, "input_iTrial_relative"=w453, "input_L_T"=w440) -> ("output_LC_Event"=w452:bool, "output_LC_Laser"=w451:bool, "output_L_Tstart"=w450:u16, "output_L_Tend"=w449:u16)  [unwired: 6 in]
        }
        frame 2 {
          w463 = u16 0
          w464 = FALSE
          # "laser2 is active"
          n194 = Index Array(array=w482, index #1=w470, index #2=w469, index #3=w468, index #4=w467, index #5=w466, index #6=w465) -> (element #1=w477:u16, element #3=w478:u16, element #4=w479:u16, element #5=w480:u16, element #6=w481:u16)  [unwired: 1 out]
          n195 = call "BRig_RT__Case_Exp__State_initTrial__LC.vi"("input_L_OnOff"=w477, "input_L_Block"=w461, "input_L_Count"=w478, "input_L_Prob"=w479, "input_L_Tdelay"=w480, "input_L_delayOpt"=w481, "input_T_state"=w476, "input_iSpout"=w461, "input_iTrial_relative"=w475, "input_L_T"=w462) -> ("output_LC_Event"=w472:bool, "output_LC_Laser"=w474:bool, "output_L_Tstart"=w473:u16, "output_L_Tend"=w471:u16)  [unwired: 6 in]
        }
        frame 3 {
          # "laser1 and laser2 are active"
          n196 = Index Array(array=w518, index #1=w497, index #2=w496, index #3=w495, index #4=w494, index #5=w493, index #6=w492, index #7=w491, index #8=w490, index #9=w489, index #10=w488, index #11=w487, index #12=w486) -> (element #1=w517:u16, element #3=w516:u16, element #4=w515:u16, element #5=w514:u16, element #6=w513:u16, element #7=w508:u16, element #9=w509:u16, element #10=w510:u16, element #11=w511:u16, element #12=w512:u16)  [unwired: 2 out]
          n197 = call "BRig_RT__Case_Exp__State_initTrial__LC.vi"("input_L_OnOff"=w517, "input_L_Block"=w483, "input_L_Count"=w516, "input_L_Prob"=w515, "input_L_Tdelay"=w514, "input_L_delayOpt"=w513, "input_T_state"=w507, "input_iSpout"=w483, "input_iTrial_relative"=w506, "input_L_T"=w485) -> ("output_LC_Event"=w505:bool, "output_LC_Laser"=w504:bool, "output_L_Tstart"=w503:u16, "output_L_Tend"=w502:u16)  [unwired: 6 in]
          n198 = call "BRig_RT__Case_Exp__State_initTrial__LC.vi"("input_L_OnOff"=w508, "input_L_Block"=w483, "input_L_Count"=w509, "input_L_Prob"=w510, "input_L_Tdelay"=w511, "input_L_delayOpt"=w512, "input_T_state"=w507, "input_iSpout"=w483, "input_iTrial_relative"=w506, "input_L_T"=w484) -> ("output_LC_Event"=w499:bool, "output_LC_Laser"=w501:bool, "output_L_Tstart"=w500:u16, "output_L_Tend"=w498:u16)  [unwired: 6 in]
        }
      }
      n199 = case shown="3" w68 {
        tunnel: w84 -> [_ w378 w400 w436]
        tunnel: w12 -> [_ w357 w379 w401]
        tunnel: w64 -> [_ w372 w394 w425]
        tunnel: w14 -> [_ w371 w393 w424]
        tunnel: [w355 w370 w382 w423] -> w98
        tunnel: [w355 w369 w382 w422] -> w97
        tunnel: [w356 w368 w381 w421] -> w94
        tunnel: [w356 w367 w381 w420] -> w93
        tunnel: [w355 w360 w392 w419] -> w95
        tunnel: [w356 w359 w391 w418] -> w92
        tunnel: [w355 w360 w390 w417] -> w96
        tunnel: [w356 w359 w389 w416] -> w91
        tunnel: w51 -> [_ w366 _ w415]
        tunnel: w50 -> [_ w365 _ w414]
        tunnel: w49 -> [_ w364 _ w413]
        tunnel: w48 -> [_ w363 _ w412]
        tunnel: w47 -> [_ w362 _ w411]
        tunnel: w46 -> [_ w361 _ w410]
        tunnel: w45 -> [_ _ w388 w409]
        tunnel: w44 -> [_ _ w387 w408]
        tunnel: w43 -> [_ _ w386 w407]
        tunnel: w42 -> [_ _ w385 w406]
        tunnel: w41 -> [_ _ w384 w405]
        tunnel: w40 -> [_ _ w383 w404]
        tunnel: w100 -> [_ w358 _ w403]
        tunnel: w99 -> [_ _ w380 w402]
        frame 0, Default {
          w356 = u16 0
          w355 = FALSE
          # "No active lasers"
        }
        frame 1 {
          w359 = u16 0
          w360 = FALSE
          # "laser1 is active"
          n200 = Index Array(array=w378, index #1=w366, index #2=w365, index #3=w364, index #4=w363, index #5=w362, index #6=w361) -> (element #1=w377:u16, element #3=w376:u16, element #4=w375:u16, element #5=w374:u16, element #6=w373:u16)  [unwired: 1 out]
          n201 = call "BRig_RT__Case_Exp__State_initTrial__LC.vi"("input_L_OnOff"=w377, "input_L_Block"=w357, "input_L_Count"=w376, "input_L_Prob"=w375, "input_L_Tdelay"=w374, "input_L_delayOpt"=w373, "input_T_state"=w372, "input_iSpout"=w357, "input_iTrial_relative"=w371, "input_L_T"=w358) -> ("output_LC_Event"=w370:bool, "output_LC_Laser"=w369:bool, "output_L_Tstart"=w368:u16, "output_L_Tend"=w367:u16)  [unwired: 6 in]
        }
        frame 2 {
          w381 = u16 0
          w382 = FALSE
          # "laser2 is active"
          n202 = Index Array(array=w400, index #1=w388, index #2=w387, index #3=w386, index #4=w385, index #5=w384, index #6=w383) -> (element #1=w395:u16, element #3=w396:u16, element #4=w397:u16, element #5=w398:u16, element #6=w399:u16)  [unwired: 1 out]
          n203 = call "BRig_RT__Case_Exp__State_initTrial__LC.vi"("input_L_OnOff"=w395, "input_L_Block"=w379, "input_L_Count"=w396, "input_L_Prob"=w397, "input_L_Tdelay"=w398, "input_L_delayOpt"=w399, "input_T_state"=w394, "input_iSpout"=w379, "input_iTrial_relative"=w393, "input_L_T"=w380) -> ("output_LC_Event"=w390:bool, "output_LC_Laser"=w392:bool, "output_L_Tstart"=w391:u16, "output_L_Tend"=w389:u16)  [unwired: 6 in]
        }
        frame 3 {
          # "laser1 and laser2 are active"
          n204 = Index Array(array=w436, index #1=w415, index #2=w414, index #3=w413, index #4=w412, index #5=w411, index #6=w410, index #7=w409, index #8=w408, index #9=w407, index #10=w406, index #11=w405, index #12=w404) -> (element #1=w435:u16, element #3=w434:u16, element #4=w433:u16, element #5=w432:u16, element #6=w431:u16, element #7=w426:u16, element #9=w427:u16, element #10=w428:u16, element #11=w429:u16, element #12=w430:u16)  [unwired: 2 out]
          n205 = call "BRig_RT__Case_Exp__State_initTrial__LC.vi"("input_L_OnOff"=w435, "input_L_Block"=w401, "input_L_Count"=w434, "input_L_Prob"=w433, "input_L_Tdelay"=w432, "input_L_delayOpt"=w431, "input_T_state"=w425, "input_iSpout"=w401, "input_iTrial_relative"=w424, "input_L_T"=w403) -> ("output_LC_Event"=w423:bool, "output_LC_Laser"=w422:bool, "output_L_Tstart"=w421:u16, "output_L_Tend"=w420:u16)  [unwired: 6 in]
          n206 = call "BRig_RT__Case_Exp__State_initTrial__LC.vi"("input_L_OnOff"=w426, "input_L_Block"=w401, "input_L_Count"=w427, "input_L_Prob"=w428, "input_L_Tdelay"=w429, "input_L_delayOpt"=w430, "input_T_state"=w425, "input_iSpout"=w401, "input_iTrial_relative"=w424, "input_L_T"=w402) -> ("output_LC_Event"=w417:bool, "output_LC_Laser"=w419:bool, "output_L_Tstart"=w418:u16, "output_L_Tend"=w416:u16)  [unwired: 6 in]
        }
      }
      n207 = call "BRig_dataCurrent_L_Cue_T_start_l1.vi"() -> ("outputL_Cue_T_start_l1"=w36:i32)  [unwired: 11 in]
      n208 = call "BRig_dataCurrent_L_Cue_T_end_l1.vi"() -> ("output_L_Cue_T_end_l1"=w37:i32)  [unwired: 11 in]
      n209 = call "BRig_dataCurrent_L_Cue_T_start_l2.vi"() -> ("output_L_Cue_T_start_l2"=w38:i32)  [unwired: 11 in]
      n210 = call "BRig_dataCurrent_L_Cue_T_end_l2.vi"() -> ("output_L_Cue_T_end_l2"=w39:i32)  [unwired: 11 in]
      n211 = call "BRig_dataCurrent_L_Cue2_T_start_l1.vi"() -> ("outputL_Cue2_T_start_l1"=w24:i32)  [unwired: 11 in]
      n212 = call "BRig_dataCurrent_L_Cue2_T_end_l1.vi"() -> ("output_L_Cue2_T_end_l1"=w25:i32)  [unwired: 11 in]
      n213 = call "BRig_dataCurrent_L_Cue2_T_start_l2.vi"() -> ("output_L_Cue2_T_start_l2"=w26:i32)  [unwired: 11 in]
      n214 = call "BRig_dataCurrent_L_Cue2_T_end_l2.vi"() -> ("output_L_Cue2_T_end_l2"=w27:i32)  [unwired: 11 in]
      n215 = Replace Array Subset(array=w120, new element #1=w118, index #1=w36, new element #2=w117, index #2=w37, new element #3=w116, index #3=w38, new element #4=w115, index #4=w39, new element #5=w94, index #5=w24, new element #6=w93, index #6=w25, new element #7=w92, index #7=w26, new element #8=w91, index #8=w27) -> (w119:u16[])
      n216 = call "BRig_dataTrial_L_Cue_event_I_l1.vi"() -> ("output_L_Cue_event_I_l1"=w16:i32)  [unwired: 11 in]
      n217 = call "BRig_dataTrial_L_Cue_trig_I_l1.vi"() -> ("output_L_Cue_trig_I_l1"=w17:i32)  [unwired: 11 in]
      n218 = call "BRig_dataTrial_L_Cue_event_I_l2.vi"() -> ("output_L_Cue_event_I_l2"=w18:i32)  [unwired: 11 in]
      n219 = call "BRig_dataTrial_L_Cue_trig_I_l2.vi"() -> ("output_L_Cue_trig_I_l2"=w19:i32)  [unwired: 11 in]
      n220 = call "BRig_dataTrial_L_Cue2_event_I_l1.vi"() -> ("output_L_Cue2_event_I_l1"=w20:i32)  [unwired: 11 in]
      n221 = call "BRig_dataTrial_L_Cue2_trig_I_l1.vi"() -> ("output_L_Cue2_trig_I_l1"=w21:i32)  [unwired: 11 in]
      n222 = call "BRig_dataTrial_L_Cue2_event_I_l2.vi"() -> ("output_L_Cue2_event_I_l2"=w22:i32)  [unwired: 11 in]
      n223 = call "BRig_dataTrial_L_Cue2_trig_I_l2.vi"() -> ("output_L_Cue2_trig_I_l2"=w23:i32)  [unwired: 11 in]
      n224 = call "BRig_arrTrig_L_Cue_event_l1.vi"() -> ("output_L_Cue_event_l1"=w28:i32)  [unwired: 11 in]
      n225 = call "BRig_arrTrig_L_Cue_laser_l1.vi"() -> ("output_L_Cue_laser_l1"=w29:i32)  [unwired: 11 in]
      n226 = call "BRig_arrTrig_L_Cue_event_l2.vi"() -> ("output_L_Cue_event_l2"=w30:i32)  [unwired: 11 in]
      n227 = call "BRig_arrTrig_L_Cue_laser_l2.vi"() -> ("output_L_Cue_laser_l2"=w31:i32)  [unwired: 11 in]
      n228 = call "BRig_arrTrig_L_Cue2_event_l1.vi"() -> ("output_L_Cue2_event_l1"=w32:i32)  [unwired: 11 in]
      n229 = call "BRig_arrTrig_L_Cue2_laser_l1.vi"() -> ("output_L_Cue2_laser_l1"=w33:i32)  [unwired: 11 in]
      n230 = call "BRig_arrTrig_L_Cue2_event_l2.vi"() -> ("output_L_Cue2_event_l2"=w34:i32)  [unwired: 11 in]
      n231 = call "BRig_arrTrig_L_Cue2_laser_l2.vi"() -> ("output_L_Cue2_laser_l2"=w35:i32)  [unwired: 11 in]
      n232 = Boolean To (0,1)(Boolean=w129) -> (0, 1=w133:i16)
      n233 = Boolean To (0,1)(Boolean=w126) -> (0, 1=w132:i16)
      n234 = Boolean To (0,1)(Boolean=w124) -> (0, 1=w130:i16)
      n235 = Boolean To (0,1)(Boolean=w122) -> (0, 1=w131:i16)
      n236 = Boolean To (0,1)(Boolean=w98) -> (0, 1=w109:i16)
      n237 = Boolean To (0,1)(Boolean=w97) -> (0, 1=w108:i16)
      n238 = Boolean To (0,1)(Boolean=w96) -> (0, 1=w106:i16)
      n239 = Boolean To (0,1)(Boolean=w95) -> (0, 1=w107:i16)
      n240 = Replace Array Subset(array=w135, new element #1=w129, index #1=w28, new element #2=w126, index #2=w29, new element #3=w124, index #3=w30, new element #4=w122, index #4=w31, new element #5=w98, index #5=w32, new element #6=w97, index #6=w33, new element #7=w96, index #7=w34, new element #8=w95, index #8=w35) -> (w134:bool[])
      n241 = To Unsigned Word Integer(number=w133) -> (unsigned 16bit integer=w128:u16)
      n242 = To Unsigned Word Integer(number=w132) -> (unsigned 16bit integer=w127:u16)
      n243 = To Unsigned Word Integer(number=w130) -> (unsigned 16bit integer=w125:u16)
      n244 = To Unsigned Word Integer(number=w131) -> (unsigned 16bit integer=w123:u16)
      n245 = To Unsigned Word Integer(number=w109) -> (unsigned 16bit integer=w104:u16)
      n246 = To Unsigned Word Integer(number=w108) -> (unsigned 16bit integer=w103:u16)
      n247 = To Unsigned Word Integer(number=w106) -> (unsigned 16bit integer=w102:u16)
      n248 = To Unsigned Word Integer(number=w107) -> (unsigned 16bit integer=w101:u16)
      n249 = Replace Array Subset(array=w86, new element #1=w128, index (row) #1=w105, index (col) #1=w16, new element #2=w127, index (row) #2=w105, index (col) #2=w17, new element #3=w125, index (row) #3=w105, index (col) #3=w18, new element #4=w123, index (row) #4=w105, index (col) #4=w19, new element #5=w104, index (row) #5=w105, index (col) #5=w20, new element #6=w103, index (row) #6=w105, index (col) #6=w21, new element #7=w102, index (row) #7=w105, index (col) #7=w22, new element #8=w101, index (row) #8=w105, index (col) #8=w23) -> (w121:u16[][])
    }
    frame False {
      w612 = 0
      # "Record laser timing"
      # "Calculate laser timing"
      # "Total Time (Cue2)"
      # "Total Time (Cue)"
      # "iTrial\nrelative"
      # "Total Time (Laser 2)"
      # "Total Time (Laser 1)"
      # "Current directionality, L or R?"
      # "laser timing case (Cue2)"
      # "Determine case for\ncalculating laser timing"
      # "2) Get relative iTrial"
      # "1) If Trial Start State = PostReward,\nThen check LC_Cue_nReward"
      # "laser2 active (Cue2)?"
      # "laser1 active (Cue2)?"
      # "laser2 active (Cue)?"
      # "laser1 active (Cue)?"
      # "1) If Trial Start State = PostReward,\nThen check LC_Cue_nReward\n\n2) Get relative iTrial"
      # "Gather variables"
      # "Last trial's\niReward\n(0 = not reward)"
      # "nTrials, current block"
      # "idx dataTrial"
      # "Total Time (Cue2)"
      # "Total Time (Cue)"
      # "# PostReward Trials"
      # "Current directionality, L or R?"
      # "Have Cue2?"
      # "Total Time (Laser 2)"
      # "Total Time (Laser 1)"
      # "Calculate settings for Cue2"
      # "Calculate settings for Cue"
      # "Set laser settings for Cue and Cue2"
      # "iTrial\nrelative"
      # "laser timing case (Cue)"
      # "Trial start state\n0 (unknown)\n1 (first)\n2 (PreReward)\n3 (PostReward)"
      # "laser2 active?"
      # "laser1 active?"
      n250 = call "BRig_dataCurrent_iSpout.vi"() -> ("output_iSpout"=w643:i32)  [unwired: 11 in]
      n251 = call "BRig_dataCurrent_LaserSwitch_l1.vi"() -> ("output_LaserSwitch_l1"=w652:i32)  [unwired: 11 in]
      n252 = call "BRig_dataCurrent_LaserSwitch_l2.vi"() -> ("output_LaserSwitch_l2"=w651:i32)  [unwired: 11 in]
      n253 = call "BRig_dataCurrent_iTrial.vi"() -> ("output_iTrial"=w617:i32)  [unwired: 11 in]
      n254 = call "BRig_dataCurrent_T_Cue.vi"() -> ("output_T_Cue"=w571:i32)  [unwired: 11 in]
      n255 = call "BRig_dataCurrent_T_Cue2.vi"() -> ("output_T_Cue2"=w570:i32)  [unwired: 11 in]
      n256 = call "BRig_dataExp_L_Ttotal_l1.vi"() -> ("output_L_Ttotal_l1"=w620:i32)  [unwired: 11 in]
      n257 = call "BRig_dataExp_L_Ttotal_l2.vi"() -> ("output_L_Ttotal_l2"=w621:i32)  [unwired: 11 in]
      n258 = call "BRig_dataExp_I_Cue2.vi"() -> ("output_I_Cue2"=w596:i32)  [unwired: 11 in]
      n259 = call "BRig_dataTrial_sTrial_start.vi"() -> ("output_sTrial_start"=w648:i32)  [unwired: 11 in]
      n260 = call "BRig_dataTrial_iTrial_PostR.vi"() -> ("output_iTrial_PostR"=w618:i32)  [unwired: 11 in]
      n261 = Index Array(array=w627, index #1=w643, index #2=w652, index #3=w651, index #4=w617, index #5=w571, index #6=w570) -> (element #1=w605:u16, element #2=w650:u16, element #3=w649:u16, element #4=w584:u16, element #5=w569:u16, element #6=w568:u16)
      n262 = Index Array(array=w619, index #1=w620, index #2=w621, index #3=w596) -> (element #1=w607:u16, element #2=w606:u16, element #3=w595:u16)
      n263 = Index Array(array=w592, index (row) #1=w612, index (col) #1=w648, index (row) #2=w612, index (col) #2=w618) -> (element #1=w543:u16, element #2=w583:u16)
      n264 = Not Equal To 0?(x=w595) -> (x != 0?=w587:bool)
      n265 = call "BRig_dataTrial_iReward.vi"() -> ("output_iReward"=w593:i32)  [unwired: 11 in]
      n266 = Not Equal To 0?(x=w650) -> (x != 0?=w588:bool)
      n267 = Not Equal To 0?(x=w649) -> (x != 0?=w589:bool)
      n268 = Index Array(array=w592, index (row)=1 ("disabled index (row)"), index (col)=w593) -> (element=w591:u16)
      n269 = case shown="3" w543 {
        tunnel: w591 -> [_ _ w739]
        tunnel: w590 -> [_ _ w740]
        tunnel: w589 -> [_ w729 w732]
        tunnel: w588 -> [_ w730 w733]
        tunnel: w587 -> [_ w728 w731]
        tunnel: [w725 w730 w738] -> w581
        tunnel: [w725 w729 w737] -> w580
        tunnel: [w725 w727 w736] -> w575
        tunnel: [w725 w726 w735] -> w574
        frame 0 {
          w725 = FALSE
        }
        frame 1, Default {
          n270 = And(x=w728, y=w730) -> (x .and. y?=w727:bool)
          n271 = And(x=w729, y=w728) -> (x .and. y?=w726:bool)
        }
        frame 3 {
          w745 = i16 0 ("f")
          n272 = Boolean To (0,1)(Boolean=w733) -> (0, 1=w743:i16)
          n273 = Select(t=i16 2, s=w732, f=w745) -> (s? t:f=w744:i16)
          n274 = Select(t=i16 4, s=w731, f=w745) -> (s? t:f=w742:i16)
          n275 = Compound Arithmetic op=ADD(w743, w744, w742) -> (w741:i16)
          n276 = case shown="7" w741 {
            tunnel: w740 -> [_ w754 w765 w779 _ w804 w825 w852]
            tunnel: w739 -> [_ w753 w764 w778 _ w800 w821 w841]
            tunnel: [w748 w752 w762 w777 w790 w799 w818 w840] -> w738
            tunnel: [w748 w751 w763 w776 w790 w797 w820 w839] -> w737
            tunnel: [w748 w751 w762 w775 w790 w798 w818 w838] -> w736
            tunnel: [w748 w751 w762 w775 w790 w797 w819 w837] -> w735
            tunnel: FALSE -> [w748 w751 w762 w775 w790 w797 w818 _]
            frame 0, Default {
            }
            frame 1 {
              n277 = call "BRig_dataLC_Cue_PostR_nRew1_l1.vi"() -> ("output_Cue_PostR_nRew1_l1"=w749:i32)  [unwired: 11 in]
              n278 = call "BRig_dataLC_Cue_PostR_nRew2_l1.vi"() -> ("output_Cue_PostR_nRew2_l1"=w750:i32)  [unwired: 11 in]
              n279 = Index Array(array=w754, index #1=w749, index #2=w750) -> (element #1=w756:u16, element #2=w755:u16)
              n280 = Equal To 0?(x=w756) -> (x = 0?=w757:bool)
              n281 = Equal?(x=w756, y=w753) -> (x = y?=w758:bool)
              n282 = Equal?(x=w755, y=w753) -> (x = y?=w759:bool)
              n283 = Compound Arithmetic op=OR(w757, w758, w759) -> (w752:bool)
            }
            frame 2 {
              n284 = call "BRig_dataLC_Cue_PostR_nRew1_l2.vi"() -> ("output_Cue_PostR_nRew1_l2"=w760:i32)  [unwired: 11 in]
              n285 = call "BRig_dataLC_Cue_PostR_nRew2_l2.vi"() -> ("output_Cue_PostR_nRew2_l2"=w761:i32)  [unwired: 11 in]
              n286 = Index Array(array=w765, index #1=w760, index #2=w761) -> (element #1=w766:u16, element #2=w767:u16)
              n287 = Equal To 0?(x=w766) -> (x = 0?=w769:bool)
              n288 = Equal?(x=w766, y=w764) -> (x = y?=w768:bool)
              n289 = Equal?(x=w767, y=w764) -> (x = y?=w770:bool)
              n290 = Compound Arithmetic op=OR(w769, w768, w770) -> (w763:bool)
            }
            frame 3 {
              n291 = call "BRig_dataLC_Cue_PostR_nRew1_l1.vi"() -> ("output_Cue_PostR_nRew1_l1"=w771:i32)  [unwired: 11 in]
              n292 = call "BRig_dataLC_Cue_PostR_nRew2_l1.vi"() -> ("output_Cue_PostR_nRew2_l1"=w772:i32)  [unwired: 11 in]
              n293 = call "BRig_dataLC_Cue_PostR_nRew1_l2.vi"() -> ("output_Cue_PostR_nRew1_l2"=w773:i32)  [unwired: 11 in]
              n294 = call "BRig_dataLC_Cue_PostR_nRew2_l2.vi"() -> ("output_Cue_PostR_nRew2_l2"=w774:i32)  [unwired: 11 in]
              n295 = Index Array(array=w779, index #1=w771, index #2=w772, index #3=w773, index #4=w774) -> (element #1=w783:u16, element #2=w782:u16, element #3=w780:u16, element #4=w781:u16)
              n296 = Equal To 0?(x=w783) -> (x = 0?=w784:bool)
              n297 = Equal?(x=w783, y=w778) -> (x = y?=w785:bool)
              n298 = Equal?(x=w782, y=w778) -> (x = y?=w786:bool)
              n299 = Equal To 0?(x=w780) -> (x = 0?=w788:bool)
              n300 = Equal?(x=w780, y=w778) -> (x = y?=w787:bool)
              n301 = Equal?(x=w781, y=w778) -> (x = y?=w789:bool)
              n302 = Compound Arithmetic op=OR(w784, w785, w786) -> (w777:bool)
              n303 = Compound Arithmetic op=OR(w788, w787, w789) -> (w776:bool)
            }
            frame 4 {
            }
            frame 5 {
              n304 = call "BRig_dataLC_Cue_PostR_nRew1_l1.vi"() -> ("output_Cue_PostR_nRew1_l1"=w793:i32)  [unwired: 11 in]
              n305 = call "BRig_dataLC_Cue_PostR_nRew2_l1.vi"() -> ("output_Cue_PostR_nRew2_l1"=w794:i32)  [unwired: 11 in]
              n306 = call "BRig_dataLC_Cue2_PostR_nRew1_l1.vi"() -> ("output_Cue2_PostR_nRew1_l1"=w791:i32)  [unwired: 11 in]
              n307 = call "BRig_dataLC_Cue2_PostR_nRew2_l1.vi"() -> ("output_Cue2_PostR_nRew2_l1"=w792:i32)  [unwired: 11 in]
              n308 = Index Array(array=w804, index #1=w793, index #2=w794, index #3=w791, index #4=w792) -> (element #1=w806:u16, element #2=w805:u16, element #3=w796:u16, element #4=w795:u16)
              n309 = Equal To 0?(x=w806) -> (x = 0?=w807:bool)
              n310 = Equal?(x=w806, y=w800) -> (x = y?=w808:bool)
              n311 = Equal?(x=w805, y=w800) -> (x = y?=w809:bool)
              n312 = Equal To 0?(x=w796) -> (x = 0?=w803:bool)
              n313 = Equal?(x=w796, y=w800) -> (x = y?=w802:bool)
              n314 = Equal?(x=w795, y=w800) -> (x = y?=w801:bool)
              n315 = Compound Arithmetic op=OR(w807, w808, w809) -> (w799:bool)
              n316 = Compound Arithmetic op=OR(w803, w802, w801) -> (w798:bool)
            }
            frame 6 {
              n317 = call "BRig_dataLC_Cue_PostR_nRew1_l2.vi"() -> ("output_Cue_PostR_nRew1_l2"=w813:i32)  [unwired: 11 in]
              n318 = call "BRig_dataLC_Cue_PostR_nRew2_l2.vi"() -> ("output_Cue_PostR_nRew2_l2"=w812:i32)  [unwired: 11 in]
              n319 = call "BRig_dataLC_Cue2_PostR_nRew1_l2.vi"() -> ("output_Cue2_PostR_nRew1_l2"=w811:i32)  [unwired: 11 in]
              n320 = call "BRig_dataLC_Cue2_PostR_nRew2_l2.vi"() -> ("output_Cue2_PostR_nRew2_l2"=w810:i32)  [unwired: 11 in]
              n321 = Index Array(array=w825, index #1=w813, index #2=w812, index #3=w811, index #4=w810) -> (element #1=w817:u16, element #2=w816:u16, element #3=w815:u16, element #4=w814:u16)
              n322 = Equal To 0?(x=w817) -> (x = 0?=w827:bool)
              n323 = Equal?(x=w817, y=w821) -> (x = y?=w826:bool)
              n324 = Equal?(x=w816, y=w821) -> (x = y?=w828:bool)
              n325 = Equal To 0?(x=w815) -> (x = 0?=w823:bool)
              n326 = Equal?(x=w815, y=w821) -> (x = y?=w824:bool)
              n327 = Equal?(x=w814, y=w821) -> (x = y?=w822:bool)
              n328 = Compound Arithmetic op=OR(w827, w826, w828) -> (w820:bool)
              n329 = Compound Arithmetic op=OR(w823, w824, w822) -> (w819:bool)
            }
            frame 7 {
              n330 = call "BRig_dataLC_Cue_PostR_nRew1_l1.vi"() -> ("output_Cue_PostR_nRew1_l1"=w833:i32)  [unwired: 11 in]
              n331 = call "BRig_dataLC_Cue_PostR_nRew2_l1.vi"() -> ("output_Cue_PostR_nRew2_l1"=w834:i32)  [unwired: 11 in]
              n332 = call "BRig_dataLC_Cue_PostR_nRew1_l2.vi"() -> ("output_Cue_PostR_nRew1_l2"=w835:i32)  [unwired: 11 in]
              n333 = call "BRig_dataLC_Cue_PostR_nRew2_l2.vi"() -> ("output_Cue_PostR_nRew2_l2"=w836:i32)  [unwired: 11 in]
              n334 = call "BRig_dataLC_Cue2_PostR_nRew1_l1.vi"() -> ("output_Cue2_PostR_nRew1_l1"=w832:i32)  [unwired: 11 in]
              n335 = call "BRig_dataLC_Cue2_PostR_nRew2_l1.vi"() -> ("output_Cue2_PostR_nRew2_l1"=w831:i32)  [unwired: 11 in]
              n336 = call "BRig_dataLC_Cue2_PostR_nRew1_l2.vi"() -> ("output_Cue2_PostR_nRew1_l2"=w830:i32)  [unwired: 11 in]
              n337 = call "BRig_dataLC_Cue2_PostR_nRew2_l2.vi"() -> ("output_Cue2_PostR_nRew2_l2"=w829:i32)  [unwired: 11 in]
              n338 = Index Array(array=w852, index #1=w833, index #2=w834, index #3=w835, index #4=w836, index #5=w832, index #6=w831, index #7=w830, index #8=w829) -> (element #1=w856:u16, element #2=w855:u16, element #3=w853:u16, element #4=w854:u16, element #5=w845:u16, element #6=w844:u16, element #7=w842:u16, element #8=w843:u16)
              n339 = Equal To 0?(x=w856) -> (x = 0?=w857:bool)
              n340 = Equal?(x=w856, y=w841) -> (x = y?=w858:bool)
              n341 = Equal?(x=w855, y=w841) -> (x = y?=w859:bool)
              n342 = Equal To 0?(x=w853) -> (x = 0?=w861:bool)
              n343 = Equal?(x=w853, y=w841) -> (x = y?=w860:bool)
              n344 = Equal?(x=w854, y=w841) -> (x = y?=w862:bool)
              n345 = Equal To 0?(x=w845) -> (x = 0?=w851:bool)
              n346 = Equal?(x=w845, y=w841) -> (x = y?=w850:bool)
              n347 = Equal?(x=w844, y=w841) -> (x = y?=w849:bool)
              n348 = Equal To 0?(x=w842) -> (x = 0?=w847:bool)
              n349 = Equal?(x=w842, y=w841) -> (x = y?=w848:bool)
              n350 = Equal?(x=w843, y=w841) -> (x = y?=w846:bool)
              n351 = Compound Arithmetic op=OR(w857, w858, w859) -> (w840:bool)
              n352 = Compound Arithmetic op=OR(w861, w860, w862) -> (w839:bool)
              n353 = Compound Arithmetic op=OR(w851, w850, w849) -> (w838:bool)
              n354 = Compound Arithmetic op=OR(w847, w848, w846) -> (w837:bool)
            }
          }
        }
      }
      n355 = case shown="1, Default" w543 {
        tunnel: [w689 w712 w723] -> w556
        tunnel: [w690 w701 w722] -> w557
        tunnel: [w691 w702 w721] -> w558
        tunnel: [w692 w703 w720] -> w559
        tunnel: [w693 w704 w719] -> w560
        tunnel: [w694 w705 w718] -> w561
        tunnel: [w695 w711 w717] -> w562
        tunnel: [w696 w706 w716] -> w563
        tunnel: [w697 w707 w715] -> w564
        tunnel: [w698 w708 w714] -> w565
        tunnel: [w699 w709 w713] -> w566
        tunnel: [w700 w710 w724] -> w567
        frame 1, Default {
          n356 = call "BRig_dataLC_Cue_First_OnOff_l1.vi"() -> ("output_Cue_First_OnOff"=w689:i32)  [unwired: 11 in]
          n357 = call "BRig_dataLC_Cue_First_Block_l1.vi"() -> ("output_Cue_First_Block"=w690:i32)  [unwired: 11 in]
          n358 = call "BRig_dataLC_Cue_First_Count_l1.vi"() -> ("output_Cue_First_Count"=w691:i32)  [unwired: 11 in]
          n359 = call "BRig_dataLC_Cue_First_Prob_l1.vi"() -> ("output_Cue_First_Prob"=w692:i32)  [unwired: 11 in]
          n360 = call "BRig_dataLC_Cue_First_Delay_l1.vi"() -> ("output_Cue_First_Delay"=w693:i32)  [unwired: 11 in]
          n361 = call "BRig_dataLC_Cue_First_DelayOpt_l1.vi"() -> ("output_Cue_First_DelayOpt"=w694:i32)  [unwired: 11 in]
          n362 = call "BRig_dataLC_Cue_First_OnOff_l2.vi"() -> ("output_Cue_First_OnOff_l2"=w695:i32)  [unwired: 11 in]
          n363 = call "BRig_dataLC_Cue_First_Block_l2.vi"() -> ("output_Cue_First_Block_l2"=w696:i32)  [unwired: 11 in]
          n364 = call "BRig_dataLC_Cue_First_Count_l2.vi"() -> ("output_Cue_First_Count_l2"=w697:i32)  [unwired: 11 in]
          n365 = call "BRig_dataLC_Cue_First_Prob_l2.vi"() -> ("output_Cue_First_Prob_l2"=w698:i32)  [unwired: 11 in]
          n366 = call "BRig_dataLC_Cue_First_Delay_l2.vi"() -> ("output_Cue_First_Delay_l2"=w699:i32)  [unwired: 11 in]
          n367 = call "BRig_dataLC_Cue_First_DelayOpt_l2.vi"() -> ("output_Cue_First_DelayOpt_l2"=w700:i32)  [unwired: 11 in]
        }
        frame 2 {
          n368 = call "BRig_dataLC_Cue_PreR_OnOff_l1.vi"() -> ("output_Cue_PreR_OnOff"=w712:i32)  [unwired: 11 in]
          n369 = call "BRig_dataLC_Cue_PreR_Block_l1.vi"() -> ("output_Cue_PreR_Block"=w701:i32)  [unwired: 11 in]
          n370 = call "BRig_dataLC_Cue_PreR_Count_l1.vi"() -> ("output_Cue_PreR_Count"=w702:i32)  [unwired: 11 in]
          n371 = call "BRig_dataLC_Cue_PreR_Prob_l1.vi"() -> ("output_Cue_PreR_Prob"=w703:i32)  [unwired: 11 in]
          n372 = call "BRig_dataLC_Cue_PreR_Delay_l1.vi"() -> ("output_Cue_PreR_Delay"=w704:i32)  [unwired: 11 in]
          n373 = call "BRig_dataLC_Cue_PreR_DelayOpt_l1.vi"() -> ("output_Cue_PreR_DelayOpt"=w705:i32)  [unwired: 11 in]
          n374 = call "BRig_dataLC_Cue_PreR_OnOff_l2.vi"() -> ("output_Cue_PreR_OnOff_l2"=w711:i32)  [unwired: 11 in]
          n375 = call "BRig_dataLC_Cue_PreR_Block_l2.vi"() -> ("output_Cue_PreR_Block_l2"=w706:i32)  [unwired: 11 in]
          n376 = call "BRig_dataLC_Cue_PreR_Count_l2.vi"() -> ("output_Cue_PreR_Count_l2"=w707:i32)  [unwired: 11 in]
          n377 = call "BRig_dataLC_Cue_PreR_Prob_l2.vi"() -> ("output_Cue_PreR_Prob_l2"=w708:i32)  [unwired: 11 in]
          n378 = call "BRig_dataLC_Cue_PreR_Delay_l2.vi"() -> ("output_Cue_PreR_Delay_l2"=w709:i32)  [unwired: 11 in]
          n379 = call "BRig_dataLC_Cue_PreR_DelayOpt_l2.vi"() -> ("output_Cue_PreR_DelayOpt_l2"=w710:i32)  [unwired: 11 in]
        }
        frame 3 {
          n380 = call "BRig_dataLC_Cue_PostR_OnOff_l1.vi"() -> ("output_Cue_PostR_OnOff"=w723:i32)  [unwired: 11 in]
          n381 = call "BRig_dataLC_Cue_PostR_Block_l1.vi"() -> ("output_Cue_PostR_Block"=w722:i32)  [unwired: 11 in]
          n382 = call "BRig_dataLC_Cue_PostR_Count_l1.vi"() -> ("output_Cue_PostR_Count"=w721:i32)  [unwired: 11 in]
          n383 = call "BRig_dataLC_Cue_PostR_Prob_l1.vi"() -> ("output_Cue_PostR_Prob"=w720:i32)  [unwired: 11 in]
          n384 = call "BRig_dataLC_Cue_PostR_Delay_l1.vi"() -> ("output_Cue_PostR_Delay"=w719:i32)  [unwired: 11 in]
          n385 = call "BRig_dataLC_Cue_PostR_DelayOpt_l1.vi"() -> ("output_Cue_PostR_DelayOpt"=w718:i32)  [unwired: 11 in]
          n386 = call "BRig_dataLC_Cue_PostR_OnOff_l2.vi"() -> ("output_Cue_PostR_OnOff_l2"=w717:i32)  [unwired: 11 in]
          n387 = call "BRig_dataLC_Cue_PostR_Block_l2.vi"() -> ("output_Cue_PostR_Block_l2"=w716:i32)  [unwired: 11 in]
          n388 = call "BRig_dataLC_Cue_PostR_Count_l2.vi"() -> ("output_Cue_PostR_Count_l2"=w715:i32)  [unwired: 11 in]
          n389 = call "BRig_dataLC_Cue_PostR_Prob_l2.vi"() -> ("output_Cue_PostR_Prob_l2"=w714:i32)  [unwired: 11 in]
          n390 = call "BRig_dataLC_Cue_PostR_Delay_l2.vi"() -> ("output_Cue_PostR_Delay_l2"=w713:i32)  [unwired: 11 in]
          n391 = call "BRig_dataLC_Cue_PostR_DelayOpt_l2.vi"() -> ("output_Cue_PostR_DelayOpt_l2"=w724:i32)  [unwired: 11 in]
        }
      }
      n392 = case shown="3" w543 {
        tunnel: [w664 w676 w688] -> w555
        tunnel: [w663 w675 w687] -> w554
        tunnel: [w662 w674 w686] -> w553
        tunnel: [w661 w673 w685] -> w552
        tunnel: [w660 w672 w684] -> w551
        tunnel: [w659 w671 w683] -> w550
        tunnel: [w658 w670 w682] -> w549
        tunnel: [w657 w669 w681] -> w548
        tunnel: [w656 w668 w680] -> w547
        tunnel: [w655 w667 w679] -> w546
        tunnel: [w654 w666 w678] -> w545
        tunnel: [w653 w665 w677] -> w544
        frame 1, Default {
          n393 = call "BRig_dataLC_Cue2_First_OnOff_l1.vi"() -> ("output_Cue2_First_OnOff"=w664:i32)  [unwired: 11 in]
          n394 = call "BRig_dataLC_Cue2_First_Block_l1.vi"() -> ("output_Cue2_First_Block"=w663:i32)  [unwired: 11 in]
          n395 = call "BRig_dataLC_Cue2_First_Count_l1.vi"() -> ("output_Cue2_First_Count"=w662:i32)  [unwired: 11 in]
          n396 = call "BRig_dataLC_Cue2_First_Prob_l1.vi"() -> ("output_Cue2_First_Prob"=w661:i32)  [unwired: 11 in]
          n397 = call "BRig_dataLC_Cue2_First_Delay_l1.vi"() -> ("output_Cue2_First_Delay"=w660:i32)  [unwired: 11 in]
          n398 = call "BRig_dataLC_Cue2_First_DelayOpt_l1.vi"() -> ("output_Cue2_First_DelayOpt"=w659:i32)  [unwired: 11 in]
          n399 = call "BRig_dataLC_Cue2_First_OnOff_l2.vi"() -> ("output_Cue2_First_OnOff_l2"=w658:i32)  [unwired: 11 in]
          n400 = call "BRig_dataLC_Cue2_First_Block_l2.vi"() -> ("output_Cue2_First_Block_l2"=w657:i32)  [unwired: 11 in]
          n401 = call "BRig_dataLC_Cue2_First_Count_l2.vi"() -> ("output_Cue2_First_Count_l2"=w656:i32)  [unwired: 11 in]
          n402 = call "BRig_dataLC_Cue2_First_Prob_l2.vi"() -> ("output_Cue2_First_Prob_l2"=w655:i32)  [unwired: 11 in]
          n403 = call "BRig_dataLC_Cue2_First_Delay_l2.vi"() -> ("output_Cue2_First_Delay_l2"=w654:i32)  [unwired: 11 in]
          n404 = call "BRig_dataLC_Cue2_First_DelayOpt_l2.vi"() -> ("output_Cue2_First_DelayOpt_l2"=w653:i32)  [unwired: 11 in]
        }
        frame 2 {
          n405 = call "BRig_dataLC_Cue2_PreR_OnOff_l1.vi"() -> ("output_Cue2_PreR_OnOff"=w676:i32)  [unwired: 11 in]
          n406 = call "BRig_dataLC_Cue2_PreR_Block_l1.vi"() -> ("output_Cue2_PreR_Block"=w675:i32)  [unwired: 11 in]
          n407 = call "BRig_dataLC_Cue2_PreR_Count_l1.vi"() -> ("output_Cue2_PreR_Count"=w674:i32)  [unwired: 11 in]
          n408 = call "BRig_dataLC_Cue2_PreR_Prob_l1.vi"() -> ("output_Cue2_PreR_Prob"=w673:i32)  [unwired: 11 in]
          n409 = call "BRig_dataLC_Cue2_PreR_Delay_l1.vi"() -> ("output_Cue2_PreR_Delay"=w672:i32)  [unwired: 11 in]
          n410 = call "BRig_dataLC_Cue2_PreR_DelayOpt_l1.vi"() -> ("output_Cue2_PreR_DelayOpt"=w671:i32)  [unwired: 11 in]
          n411 = call "BRig_dataLC_Cue2_PreR_OnOff_l2.vi"() -> ("output_Cue2_PreR_OnOff_l2"=w670:i32)  [unwired: 11 in]
          n412 = call "BRig_dataLC_Cue2_PreR_Block_l2.vi"() -> ("output_Cue2_PreR_Block_l2"=w669:i32)  [unwired: 11 in]
          n413 = call "BRig_dataLC_Cue2_PreR_Count_l2.vi"() -> ("output_Cue2_PreR_Count_l2"=w668:i32)  [unwired: 11 in]
          n414 = call "BRig_dataLC_Cue2_PreR_Prob_l2.vi"() -> ("output_Cue2_PreR_Prob_l2"=w667:i32)  [unwired: 11 in]
          n415 = call "BRig_dataLC_Cue2_PreR_Delay_l2.vi"() -> ("output_Cue2_PreR_Delay_l2"=w666:i32)  [unwired: 11 in]
          n416 = call "BRig_dataLC_Cue2_PreR_DelayOpt_l2.vi"() -> ("output_Cue2_PreR_DelayOpt_l2"=w665:i32)  [unwired: 11 in]
        }
        frame 3 {
          n417 = call "BRig_dataLC_Cue2_PostR_OnOff_l1.vi"() -> ("output_Cue2_PostR_OnOff"=w688:i32)  [unwired: 11 in]
          n418 = call "BRig_dataLC_Cue2_PostR_Block_l1.vi"() -> ("output_Cue2_PostR_Block"=w687:i32)  [unwired: 11 in]
          n419 = call "BRig_dataLC_Cue2_PostR_Count_l1.vi"() -> ("output_Cue2_PostR_Count"=w686:i32)  [unwired: 11 in]
          n420 = call "BRig_dataLC_Cue2_PostR_Prob_l1.vi"() -> ("output_Cue2_PostR_Prob"=w685:i32)  [unwired: 11 in]
          n421 = call "BRig_dataLC_Cue2_PostR_Delay_l1.vi"() -> ("output_Cue2_PostR_Delay"=w684:i32)  [unwired: 11 in]
          n422 = call "BRig_dataLC_Cue2_PostR_DelayOpt_l1.vi"() -> ("output_Cue2_PostR_DelayOpt"=w683:i32)  [unwired: 11 in]
          n423 = call "BRig_dataLC_Cue2_PostR_OnOff_l2.vi"() -> ("output_Cue2_PostR_OnOff_l2"=w682:i32)  [unwired: 11 in]
          n424 = call "BRig_dataLC_Cue2_PostR_Block_l2.vi"() -> ("output_Cue2_PostR_Block_l2"=w681:i32)  [unwired: 11 in]
          n425 = call "BRig_dataLC_Cue2_PostR_Count_l2.vi"() -> ("output_Cue2_PostR_Count_l2"=w680:i32)  [unwired: 11 in]
          n426 = call "BRig_dataLC_Cue2_PostR_Prob_l2.vi"() -> ("output_Cue2_PostR_Prob_l2"=w679:i32)  [unwired: 11 in]
          n427 = call "BRig_dataLC_Cue2_PostR_Delay_l2.vi"() -> ("output_Cue2_PostR_Delay_l2"=w678:i32)  [unwired: 11 in]
          n428 = call "BRig_dataLC_Cue2_PostR_DelayOpt_l2.vi"() -> ("output_Cue2_PostR_DelayOpt_l2"=w677:i32)  [unwired: 11 in]
        }
      }
      n429 = Less?(x=w543, y=u16 3) -> (x < y?=w585:bool)
      n430 = Select(t=w584, s=w585, f=w583) -> (s? t:f=w582:u16)
      n431 = Boolean To (0,1)(Boolean=w581) -> (0, 1=w645:i16)
      n432 = Boolean To (0,1)(Boolean=w575) -> (0, 1=w578:i16)
      n433 = Select(t=i16 2, s=w580, f=i16 0) -> (s? t:f=w646:i16)
      n434 = Select(t=i16 2, s=w574, f=i16 0) -> (s? t:f=w577:i16)
      n435 = Add(x=w645, y=w646) -> (x+y=w573:i16)
      n436 = Add(x=w578, y=w577) -> (x+y=w572:i16)
      n437 = case shown="2" w573 {
        tunnel: w590 -> [_ w985 w1008 w1046]
        tunnel: w605 -> [_ w977 w1000 w1032]
        tunnel: w569 -> [_ w978 w1001 w1033]
        tunnel: w582 -> [_ w976 w999 w1031]
        tunnel: [w955 w975 w988 w1030] -> w636
        tunnel: [w955 w974 w988 w1029] -> w633
        tunnel: [w956 w973 w987 w1028] -> w625
        tunnel: [w956 w972 w987 w1027] -> w624
        tunnel: [w955 w959 w998 w1026] -> w629
        tunnel: [w956 w958 w997 w1025] -> w623
        tunnel: [w955 w959 w996 w1024] -> w631
        tunnel: [w956 w958 w995 w1023] -> w622
        tunnel: w556 -> [_ w971 _ w1022]
        tunnel: w557 -> [_ w970 _ w1021]
        tunnel: w558 -> [_ w969 _ w1020]
        tunnel: w559 -> [_ w968 _ w1019]
        tunnel: w560 -> [_ w967 _ w1018]
        tunnel: w561 -> [_ w966 _ w1017]
        tunnel: w562 -> [_ w965 w994 w1016]
        tunnel: w563 -> [_ w964 w993 w1015]
        tunnel: w564 -> [_ w963 w992 w1014]
        tunnel: w565 -> [_ w962 w991 w1013]
        tunnel: w566 -> [_ w961 w990 w1012]
        tunnel: w567 -> [_ w960 w989 w1011]
        tunnel: w607 -> [_ w957 _ w1010]
        tunnel: w606 -> [_ _ w986 w1009]
        frame 0, Default {
          w956 = u16 0
          w955 = FALSE
          # "No active lasers"
        }
        frame 1 {
          w958 = u16 0
          w959 = FALSE
          # "laser1 is active"
          n438 = Index Array(array=w985, index #1=w971, index #2=w970, index #3=w969, index #4=w968, index #5=w967, index #6=w966, index #7=w965, index #8=w964, index #9=w963, index #10=w962, index #11=w961, index #12=w960) -> (element #1=w984:u16, element #2=w983:u16, element #3=w982:u16, element #4=w981:u16, element #5=w980:u16, element #6=w979:u16)  [unwired: 6 out]
          n439 = call "BRig_RT__Case_Exp__State_initTrial__LC.vi"("input_L_OnOff"=w984, "input_L_Block"=w983, "input_L_Count"=w982, "input_L_Prob"=w981, "input_L_Tdelay"=w980, "input_L_delayOpt"=w979, "input_T_state"=w978, "input_iSpout"=w977, "input_iTrial_relative"=w976, "input_L_T"=w957) -> ("output_LC_Event"=w975:bool, "output_LC_Laser"=w974:bool, "output_L_Tstart"=w973:u16, "output_L_Tend"=w972:u16)  [unwired: 6 in]
        }
        frame 2 {
          w987 = u16 0
          w988 = FALSE
          # "laser2 is active"
          n440 = Index Array(array=w1008, index #1=w994, index #2=w993, index #3=w992, index #4=w991, index #5=w990, index #6=w989) -> (element #1=w1002:u16, element #2=w1003:u16, element #3=w1004:u16, element #4=w1005:u16, element #5=w1006:u16, element #6=w1007:u16)
          n441 = call "BRig_RT__Case_Exp__State_initTrial__LC.vi"("input_L_OnOff"=w1002, "input_L_Block"=w1003, "input_L_Count"=w1004, "input_L_Prob"=w1005, "input_L_Tdelay"=w1006, "input_L_delayOpt"=w1007, "input_T_state"=w1001, "input_iSpout"=w1000, "input_iTrial_relative"=w999, "input_L_T"=w986) -> ("output_LC_Event"=w996:bool, "output_LC_Laser"=w998:bool, "output_L_Tstart"=w997:u16, "output_L_Tend"=w995:u16)  [unwired: 6 in]
        }
        frame 3 {
          # "laser1 and laser2 are active"
          n442 = Index Array(array=w1046, index #1=w1022, index #2=w1021, index #3=w1020, index #4=w1019, index #5=w1018, index #6=w1017, index #7=w1016, index #8=w1015, index #9=w1014, index #10=w1013, index #11=w1012, index #12=w1011) -> (element #1=w1045:u16, element #2=w1044:u16, element #3=w1043:u16, element #4=w1042:u16, element #5=w1041:u16, element #6=w1040:u16, element #7=w1034:u16, element #8=w1035:u16, element #9=w1036:u16, element #10=w1037:u16, element #11=w1038:u16, element #12=w1039:u16)
          n443 = call "BRig_RT__Case_Exp__State_initTrial__LC.vi"("input_L_OnOff"=w1045, "input_L_Block"=w1044, "input_L_Count"=w1043, "input_L_Prob"=w1042, "input_L_Tdelay"=w1041, "input_L_delayOpt"=w1040, "input_T_state"=w1033, "input_iSpout"=w1032, "input_iTrial_relative"=w1031, "input_L_T"=w1010) -> ("output_LC_Event"=w1030:bool, "output_LC_Laser"=w1029:bool, "output_L_Tstart"=w1028:u16, "output_L_Tend"=w1027:u16)  [unwired: 6 in]
          n444 = call "BRig_RT__Case_Exp__State_initTrial__LC.vi"("input_L_OnOff"=w1034, "input_L_Block"=w1035, "input_L_Count"=w1036, "input_L_Prob"=w1037, "input_L_Tdelay"=w1038, "input_L_delayOpt"=w1039, "input_T_state"=w1033, "input_iSpout"=w1032, "input_iTrial_relative"=w1031, "input_L_T"=w1009) -> ("output_LC_Event"=w1024:bool, "output_LC_Laser"=w1026:bool, "output_L_Tstart"=w1025:u16, "output_L_Tend"=w1023:u16)  [unwired: 6 in]
        }
      }
      n445 = case shown="3" w572 {
        tunnel: w590 -> [_ w893 w916 w954]
        tunnel: w605 -> [_ w885 w908 w940]
        tunnel: w568 -> [_ w886 w909 w941]
        tunnel: w582 -> [_ w884 w907 w939]
        tunnel: [w863 w883 w896 w938] -> w604
        tunnel: [w863 w882 w896 w937] -> w603
        tunnel: [w864 w881 w895 w936] -> w600
        tunnel: [w864 w880 w895 w935] -> w599
        tunnel: [w863 w867 w906 w934] -> w601
        tunnel: [w864 w866 w905 w933] -> w598
        tunnel: [w863 w867 w904 w932] -> w602
        tunnel: [w864 w866 w903 w931] -> w597
        tunnel: w555 -> [_ w879 _ w930]
        tunnel: w554 -> [_ w878 _ w929]
        tunnel: w553 -> [_ w877 _ w928]
        tunnel: w552 -> [_ w876 _ w927]
        tunnel: w551 -> [_ w875 _ w926]
        tunnel: w550 -> [_ w874 _ w925]
        tunnel: w549 -> [_ w873 w902 w924]
        tunnel: w548 -> [_ w872 w901 w923]
        tunnel: w547 -> [_ w871 w900 w922]
        tunnel: w546 -> [_ w870 w899 w921]
        tunnel: w545 -> [_ w869 w898 w920]
        tunnel: w544 -> [_ w868 w897 w919]
        tunnel: w607 -> [_ w865 _ w918]
        tunnel: w606 -> [_ _ w894 w917]
        frame 0, Default {
          w864 = u16 0
          w863 = FALSE
          # "No active lasers"
        }
        frame 1 {
          w866 = u16 0
          w867 = FALSE
          # "laser1 is active"
          n446 = Index Array(array=w893, index #1=w879, index #2=w878, index #3=w877, index #4=w876, index #5=w875, index #6=w874, index #7=w873, index #8=w872, index #9=w871, index #10=w870, index #11=w869, index #12=w868) -> (element #1=w892:u16, element #2=w891:u16, element #3=w890:u16, element #4=w889:u16, element #5=w888:u16, element #6=w887:u16)  [unwired: 6 out]
          n447 = call "BRig_RT__Case_Exp__State_initTrial__LC.vi"("input_L_OnOff"=w892, "input_L_Block"=w891, "input_L_Count"=w890, "input_L_Prob"=w889, "input_L_Tdelay"=w888, "input_L_delayOpt"=w887, "input_T_state"=w886, "input_iSpout"=w885, "input_iTrial_relative"=w884, "input_L_T"=w865) -> ("output_LC_Event"=w883:bool, "output_LC_Laser"=w882:bool, "output_L_Tstart"=w881:u16, "output_L_Tend"=w880:u16)  [unwired: 6 in]
        }
        frame 2 {
          w895 = u16 0
          w896 = FALSE
          # "laser2 is active"
          n448 = Index Array(array=w916, index #1=w902, index #2=w901, index #3=w900, index #4=w899, index #5=w898, index #6=w897) -> (element #1=w910:u16, element #2=w911:u16, element #3=w912:u16, element #4=w913:u16, element #5=w914:u16, element #6=w915:u16)
          n449 = call "BRig_RT__Case_Exp__State_initTrial__LC.vi"("input_L_OnOff"=w910, "input_L_Block"=w911, "input_L_Count"=w912, "input_L_Prob"=w913, "input_L_Tdelay"=w914, "input_L_delayOpt"=w915, "input_T_state"=w909, "input_iSpout"=w908, "input_iTrial_relative"=w907, "input_L_T"=w894) -> ("output_LC_Event"=w904:bool, "output_LC_Laser"=w906:bool, "output_L_Tstart"=w905:u16, "output_L_Tend"=w903:u16)  [unwired: 6 in]
        }
        frame 3 {
          # "laser1 and laser2 are active"
          n450 = Index Array(array=w954, index #1=w930, index #2=w929, index #3=w928, index #4=w927, index #5=w926, index #6=w925, index #7=w924, index #8=w923, index #9=w922, index #10=w921, index #11=w920, index #12=w919) -> (element #1=w953:u16, element #2=w952:u16, element #3=w951:u16, element #4=w950:u16, element #5=w949:u16, element #6=w948:u16, element #7=w942:u16, element #8=w943:u16, element #9=w944:u16, element #10=w945:u16, element #11=w946:u16, element #12=w947:u16)
          n451 = call "BRig_RT__Case_Exp__State_initTrial__LC.vi"("input_L_OnOff"=w953, "input_L_Block"=w952, "input_L_Count"=w951, "input_L_Prob"=w950, "input_L_Tdelay"=w949, "input_L_delayOpt"=w948, "input_T_state"=w941, "input_iSpout"=w940, "input_iTrial_relative"=w939, "input_L_T"=w918) -> ("output_LC_Event"=w938:bool, "output_LC_Laser"=w937:bool, "output_L_Tstart"=w936:u16, "output_L_Tend"=w935:u16)  [unwired: 6 in]
          n452 = call "BRig_RT__Case_Exp__State_initTrial__LC.vi"("input_L_OnOff"=w942, "input_L_Block"=w943, "input_L_Count"=w944, "input_L_Prob"=w945, "input_L_Tdelay"=w946, "input_L_delayOpt"=w947, "input_T_state"=w941, "input_iSpout"=w940, "input_iTrial_relative"=w939, "input_L_T"=w917) -> ("output_LC_Event"=w932:bool, "output_LC_Laser"=w934:bool, "output_L_Tstart"=w933:u16, "output_L_Tend"=w931:u16)  [unwired: 6 in]
        }
      }
      n453 = call "BRig_dataCurrent_L_Cue_T_start_l1.vi"() -> ("outputL_Cue_T_start_l1"=w539:i32)  [unwired: 11 in]
      n454 = call "BRig_dataCurrent_L_Cue_T_end_l1.vi"() -> ("output_L_Cue_T_end_l1"=w540:i32)  [unwired: 11 in]
      n455 = call "BRig_dataCurrent_L_Cue_T_start_l2.vi"() -> ("output_L_Cue_T_start_l2"=w541:i32)  [unwired: 11 in]
      n456 = call "BRig_dataCurrent_L_Cue_T_end_l2.vi"() -> ("output_L_Cue_T_end_l2"=w542:i32)  [unwired: 11 in]
      n457 = call "BRig_dataCurrent_L_Cue2_T_start_l1.vi"() -> ("outputL_Cue2_T_start_l1"=w527:i32)  [unwired: 11 in]
      n458 = call "BRig_dataCurrent_L_Cue2_T_end_l1.vi"() -> ("output_L_Cue2_T_end_l1"=w528:i32)  [unwired: 11 in]
      n459 = call "BRig_dataCurrent_L_Cue2_T_start_l2.vi"() -> ("output_L_Cue2_T_start_l2"=w529:i32)  [unwired: 11 in]
      n460 = call "BRig_dataCurrent_L_Cue2_T_end_l2.vi"() -> ("output_L_Cue2_T_end_l2"=w530:i32)  [unwired: 11 in]
      n461 = Replace Array Subset(array=w627, new element #1=w625, index #1=w539, new element #2=w624, index #2=w540, new element #3=w623, index #3=w541, new element #4=w622, index #4=w542, new element #5=w600, index #5=w527, new element #6=w599, index #6=w528, new element #7=w598, index #7=w529, new element #8=w597, index #8=w530) -> (w626:u16[])
      n462 = call "BRig_dataTrial_L_Cue_event_I_l1.vi"() -> ("output_L_Cue_event_I_l1"=w519:i32)  [unwired: 11 in]
      n463 = call "BRig_dataTrial_L_Cue_trig_I_l1.vi"() -> ("output_L_Cue_trig_I_l1"=w520:i32)  [unwired: 11 in]
      n464 = call "BRig_dataTrial_L_Cue_event_I_l2.vi"() -> ("output_L_Cue_event_I_l2"=w521:i32)  [unwired: 11 in]
      n465 = call "BRig_dataTrial_L_Cue_trig_I_l2.vi"() -> ("output_L_Cue_trig_I_l2"=w522:i32)  [unwired: 11 in]
      n466 = call "BRig_dataTrial_L_Cue2_event_I_l1.vi"() -> ("output_L_Cue2_event_I_l1"=w523:i32)  [unwired: 11 in]
      n467 = call "BRig_dataTrial_L_Cue2_trig_I_l1.vi"() -> ("output_L_Cue2_trig_I_l1"=w524:i32)  [unwired: 11 in]
      n468 = call "BRig_dataTrial_L_Cue2_event_I_l2.vi"() -> ("output_L_Cue2_event_I_l2"=w525:i32)  [unwired: 11 in]
      n469 = call "BRig_dataTrial_L_Cue2_trig_I_l2.vi"() -> ("output_L_Cue2_trig_I_l2"=w526:i32)  [unwired: 11 in]
      n470 = call "BRig_arrTrig_L_Cue_event_l1.vi"() -> ("output_L_Cue_event_l1"=w531:i32)  [unwired: 11 in]
      n471 = call "BRig_arrTrig_L_Cue_laser_l1.vi"() -> ("output_L_Cue_laser_l1"=w532:i32)  [unwired: 11 in]
      n472 = call "BRig_arrTrig_L_Cue_event_l2.vi"() -> ("output_L_Cue_event_l2"=w533:i32)  [unwired: 11 in]
      n473 = call "BRig_arrTrig_L_Cue_laser_l2.vi"() -> ("output_L_Cue_laser_l2"=w534:i32)  [unwired: 11 in]
      n474 = call "BRig_arrTrig_L_Cue2_event_l1.vi"() -> ("output_L_Cue2_event_l1"=w535:i32)  [unwired: 11 in]
      n475 = call "BRig_arrTrig_L_Cue2_laser_l1.vi"() -> ("output_L_Cue2_laser_l1"=w536:i32)  [unwired: 11 in]
      n476 = call "BRig_arrTrig_L_Cue2_event_l2.vi"() -> ("output_L_Cue2_event_l2"=w537:i32)  [unwired: 11 in]
      n477 = call "BRig_arrTrig_L_Cue2_laser_l2.vi"() -> ("output_L_Cue2_laser_l2"=w538:i32)  [unwired: 11 in]
      n478 = Boolean To (0,1)(Boolean=w636) -> (0, 1=w640:i16)
      n479 = Boolean To (0,1)(Boolean=w633) -> (0, 1=w639:i16)
      n480 = Boolean To (0,1)(Boolean=w631) -> (0, 1=w637:i16)
      n481 = Boolean To (0,1)(Boolean=w629) -> (0, 1=w638:i16)
      n482 = Boolean To (0,1)(Boolean=w604) -> (0, 1=w616:i16)
      n483 = Boolean To (0,1)(Boolean=w603) -> (0, 1=w615:i16)
      n484 = Boolean To (0,1)(Boolean=w602) -> (0, 1=w613:i16)
      n485 = Boolean To (0,1)(Boolean=w601) -> (0, 1=w614:i16)
      n486 = Replace Array Subset(array=w642, new element #1=w636, index #1=w531, new element #2=w633, index #2=w532, new element #3=w631, index #3=w533, new element #4=w629, index #4=w534, new element #5=w604, index #5=w535, new element #6=w603, index #6=w536, new element #7=w602, index #7=w537, new element #8=w601, index #8=w538) -> (w641:bool[])
      n487 = To Unsigned Word Integer(number=w640) -> (unsigned 16bit integer=w635:u16)
      n488 = To Unsigned Word Integer(number=w639) -> (unsigned 16bit integer=w634:u16)
      n489 = To Unsigned Word Integer(number=w637) -> (unsigned 16bit integer=w632:u16)
      n490 = To Unsigned Word Integer(number=w638) -> (unsigned 16bit integer=w630:u16)
      n491 = To Unsigned Word Integer(number=w616) -> (unsigned 16bit integer=w611:u16)
      n492 = To Unsigned Word Integer(number=w615) -> (unsigned 16bit integer=w610:u16)
      n493 = To Unsigned Word Integer(number=w613) -> (unsigned 16bit integer=w609:u16)
      n494 = To Unsigned Word Integer(number=w614) -> (unsigned 16bit integer=w608:u16)
      n495 = Replace Array Subset(array=w592, new element #1=w635, index (row) #1=w612, index (col) #1=w519, new element #2=w634, index (row) #2=w612, index (col) #2=w520, new element #3=w632, index (row) #3=w612, index (col) #3=w521, new element #4=w630, index (row) #4=w612, index (col) #4=w522, new element #5=w611, index (row) #5=w612, index (col) #5=w523, new element #6=w610, index (row) #6=w612, index (col) #6=w524, new element #7=w609, index (row) #7=w612, index (col) #7=w525, new element #8=w608, index (row) #8=w612, index (col) #8=w526) -> (w628:u16[][])
    }
  }
  "output_dataCurrent" <- w7
  "output_arrTrig" <- w10
  "output_dataTrial" <- w9
